vi "Hysteresis.vi"(0 "Max":dbl=4.0 min=-5.0 max=5.0 format="%.3f", 1 "Min":dbl=-4.0 min=-5.0 max=5.0 format="%.3f", 2 "?":bool, 3 "SubVI":bool, 4 "Pattern":string(combo)="0", 5 "?":bool, 6 "Min":dbl=-4.0 min=-10.5 max=10.5 format="%.3f", 7 "Max":dbl=4.0 min=-10.5 max=10.5 format="%.3f", 8 "Amplitude":dbl=2.0 min=1e-09 max=2.0 format="%.3f", 10 "Frequency":dbl=4.0 min=0.001 max=2500000.0 format="%.3g", 13 "?":bool, 14 "Loop":dbl=1.0 min=1.0 step=1.0 format="%#_4g", 16 "Steps":dbl=15.0 min=1.0 step=1.0 format="%#_4g", 18 "Bias Time":dbl=1.0 min=0.0 format="%.4f") -> (12 "Total Loop Time":dbl=40.0 min=0.0 format="%.4f")   [LabVIEW 2016]
uses:
  <vilib>/Utility/file.llb/Write Delimited Spreadsheet (DBL).vi
  <instrlib>/Stanford Research SR865/Stanford Research SR865.lvlib
panel:
  in  "Save As Path":path
  in  "Save As Path":path
  in  "Save As Path":path
  in  "Save As Path":path
  in  "Save As Path":path
  in  "Save As Path":path
  in  "Save As Path":path
  out "Output3-Time":cluster{dbl[], dbl[]}(graph)
  out "Output3-Potential Difference":cluster{dbl[], dbl[]}(graph)
  out "Output2-Time":cluster{dbl[], dbl[]}(graph)
  out "Potential Difference-Time":cluster{dbl[], dbl[]}(graph)
  out "Output1-Time":cluster{dbl[], dbl[]}(graph)
  out "Output1-Potential Difference":cluster{dbl[], dbl[]}(graph)
  out "Output2-Potential Difference":cluster{dbl[], dbl[]}(graph)
  in  "Output 3":i32(ring) items=["None"=-1, "X output"=0, "Y output"=1, "R output"=2, "Theta output"=3, "Aux In 1"=4, "Aux In 2"=5, "Aux In 3"=6, "Aux In 4"=7, "Aux Out 1"=8, "Aux Out 2"=9, "Xnoise"=10, "Ynoise"=11, "Reference Phase"=12, "Sine Out Amplitude"=13, "DC Level"=14, "Int. Ref. Frequency"=15, "Ext. Ref. Frequency"=16]
  in  "Aux Channel":u16(ring)=1 items=["Aux Output 1"=1, "Aux Output 2"=2, "Aux Output 3"=3, "Aux Output 4"=4]
  in  "Output 2":i32(ring)=3 items=["X output", "Y output", "R output", "Theta output", "Aux In 1", "Aux In 2", "Aux In 3", "Aux In 4", "Aux Out 1", "Aux Out 2", "Xnoise", "Ynoise", "Reference Phase", "Sine Out Amplitude", "DC Level", "Int. Ref. Frequency", "Ext. Ref. Frequency"]
  in  "Output 1":i32(ring)=2 items=["X output", "Y output", "R output", "Theta output", "Aux In 1", "Aux In 2", "Aux In 3", "Aux In 4", "Aux Out 1", "Aux Out 2", "Xnoise", "Ynoise", "Reference Phase", "Sine Out Amplitude", "DC Level", "Int. Ref. Frequency", "Ext. Ref. Frequency"]
  in  "Bias Intermission":dbl=0.25 min=0.0 format="%.4f"
  in  "0 V Intermission":dbl=0.25 min=0.0 format="%.4f"
  in  "0 V Time":dbl=1.0 min=0.0 format="%.4f"
  out "VISA resource name out":refnum<visa-resource-name>
  out "error out":errorcluster
  in  "VISA resource name":refnum<visa-resource-name>="LIA"
  in  "error in (no error)":errorcluster
  out "Step Time":dbl=2.5 format="%#.4g"
  # "Configure"
  # "Sine Out DC"
  # "V"
  # "V"
  # "Sine Out AC"
  # "V"
  # "Hz"
  # "Aux Out DC Sawtooth"
  # "V"
  # "V"
  # "Times"
  # "times"
  # "s"
  # "s"
  # "s"
  # "s"
  # "s"
  # "s"
  # "Outputs"
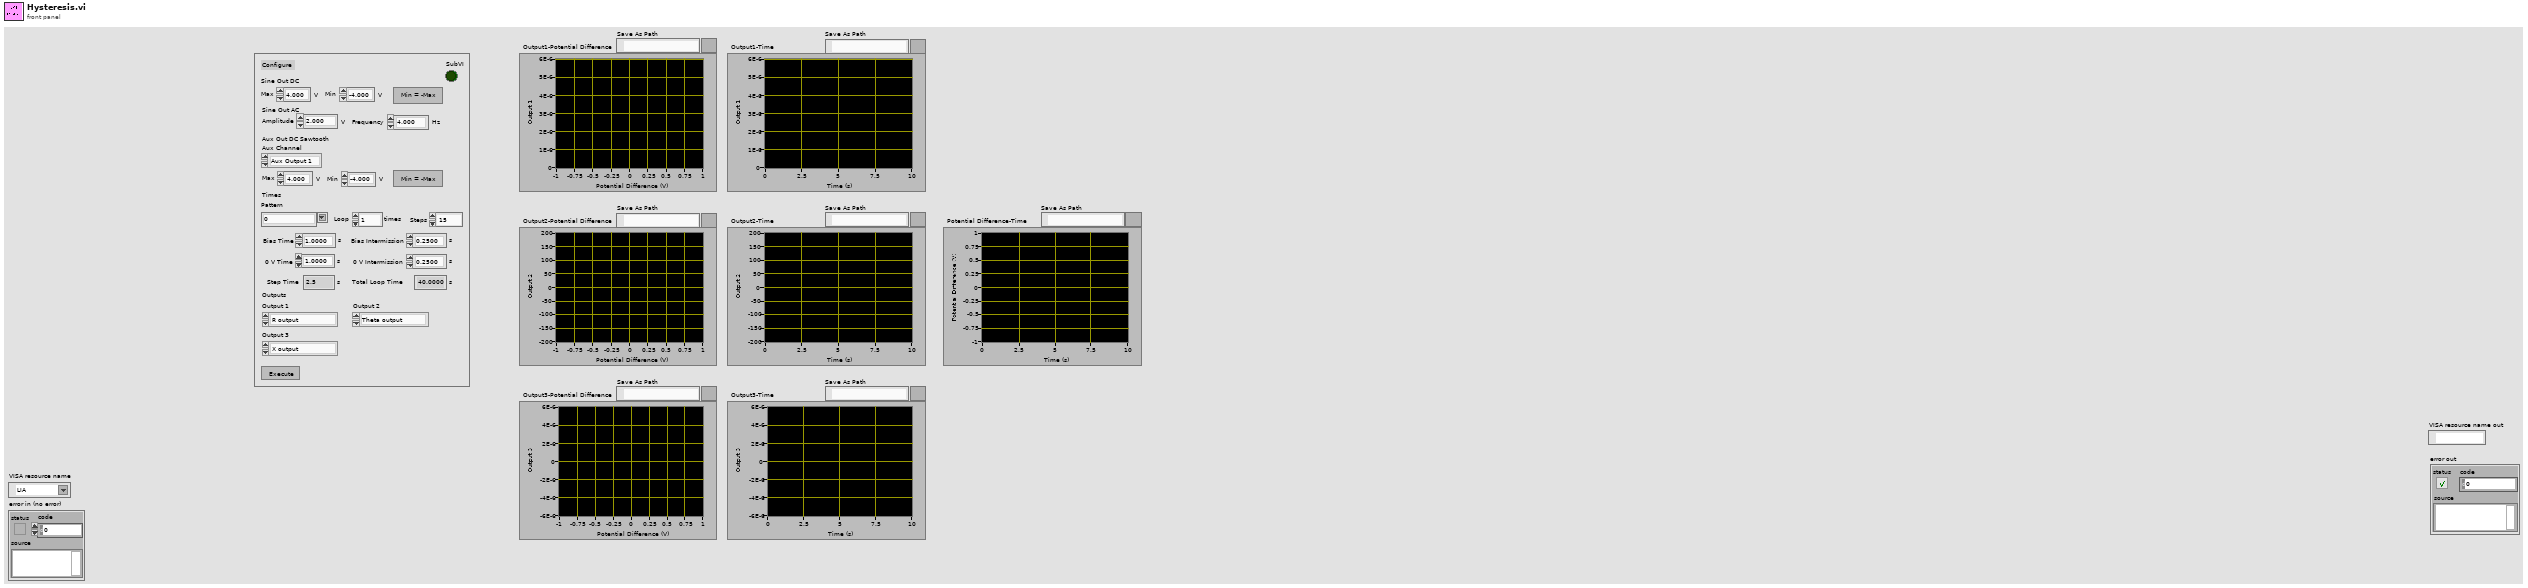
[diagram p1: front panel]
types:
  T1 = cluster{"Value 1":dbl, "Value 2":dbl, "Value 3":dbl}
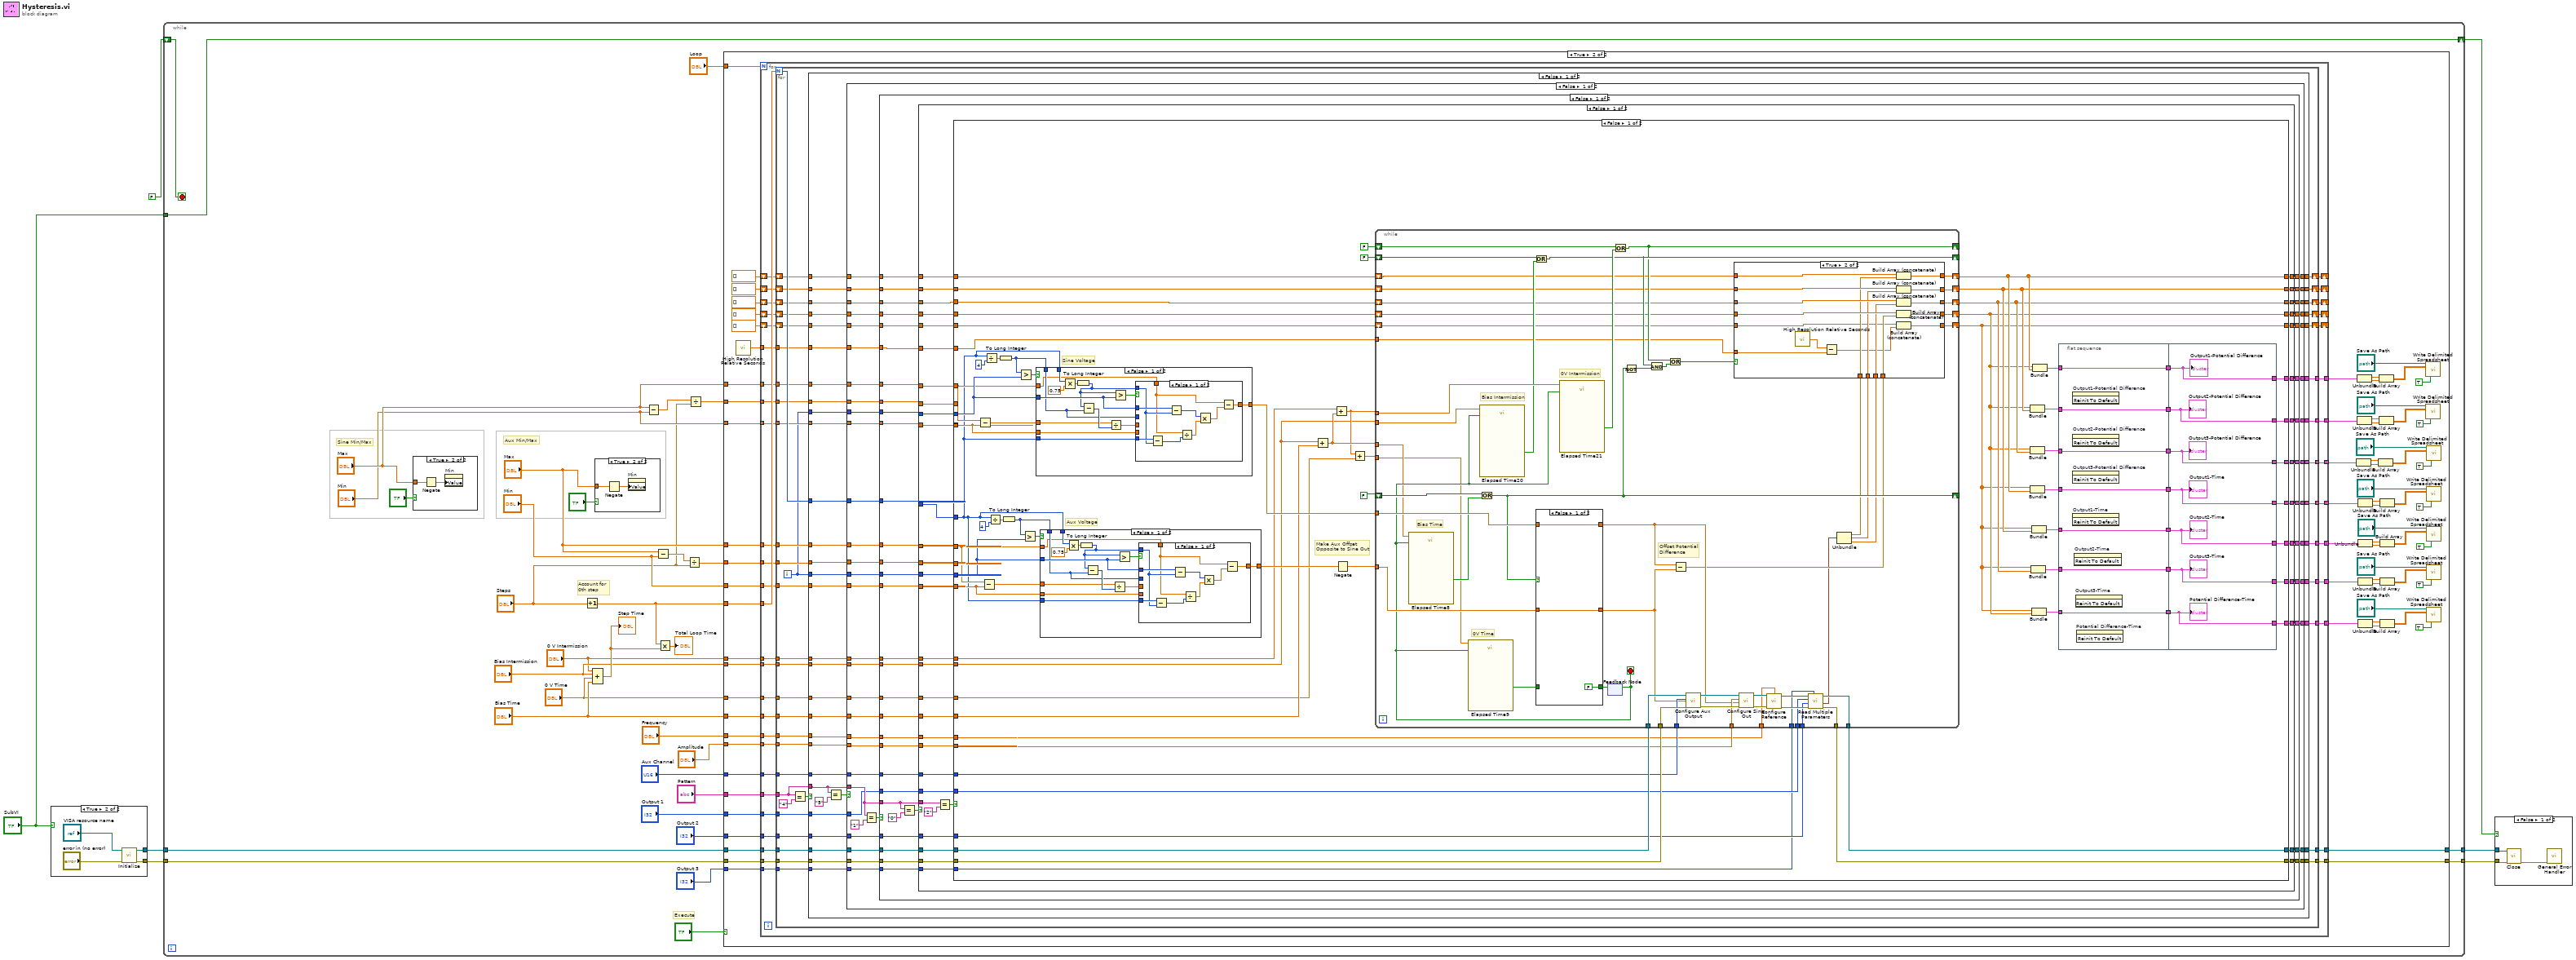
[diagram p0: block diagram]
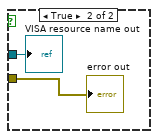
[diagram p2: hidden frame]
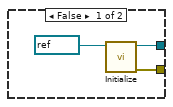
[diagram p3: hidden frame]
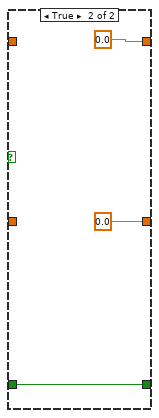
[diagram p6: hidden frame]
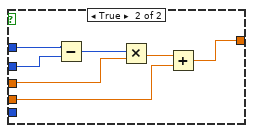
[diagram p7: hidden frame]
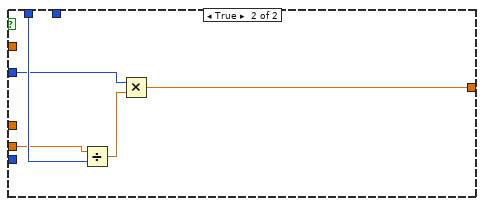
[diagram p8: hidden frame]
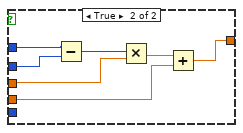
[diagram p9: hidden frame]
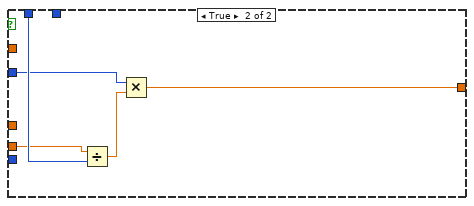
[diagram p10: hidden frame]
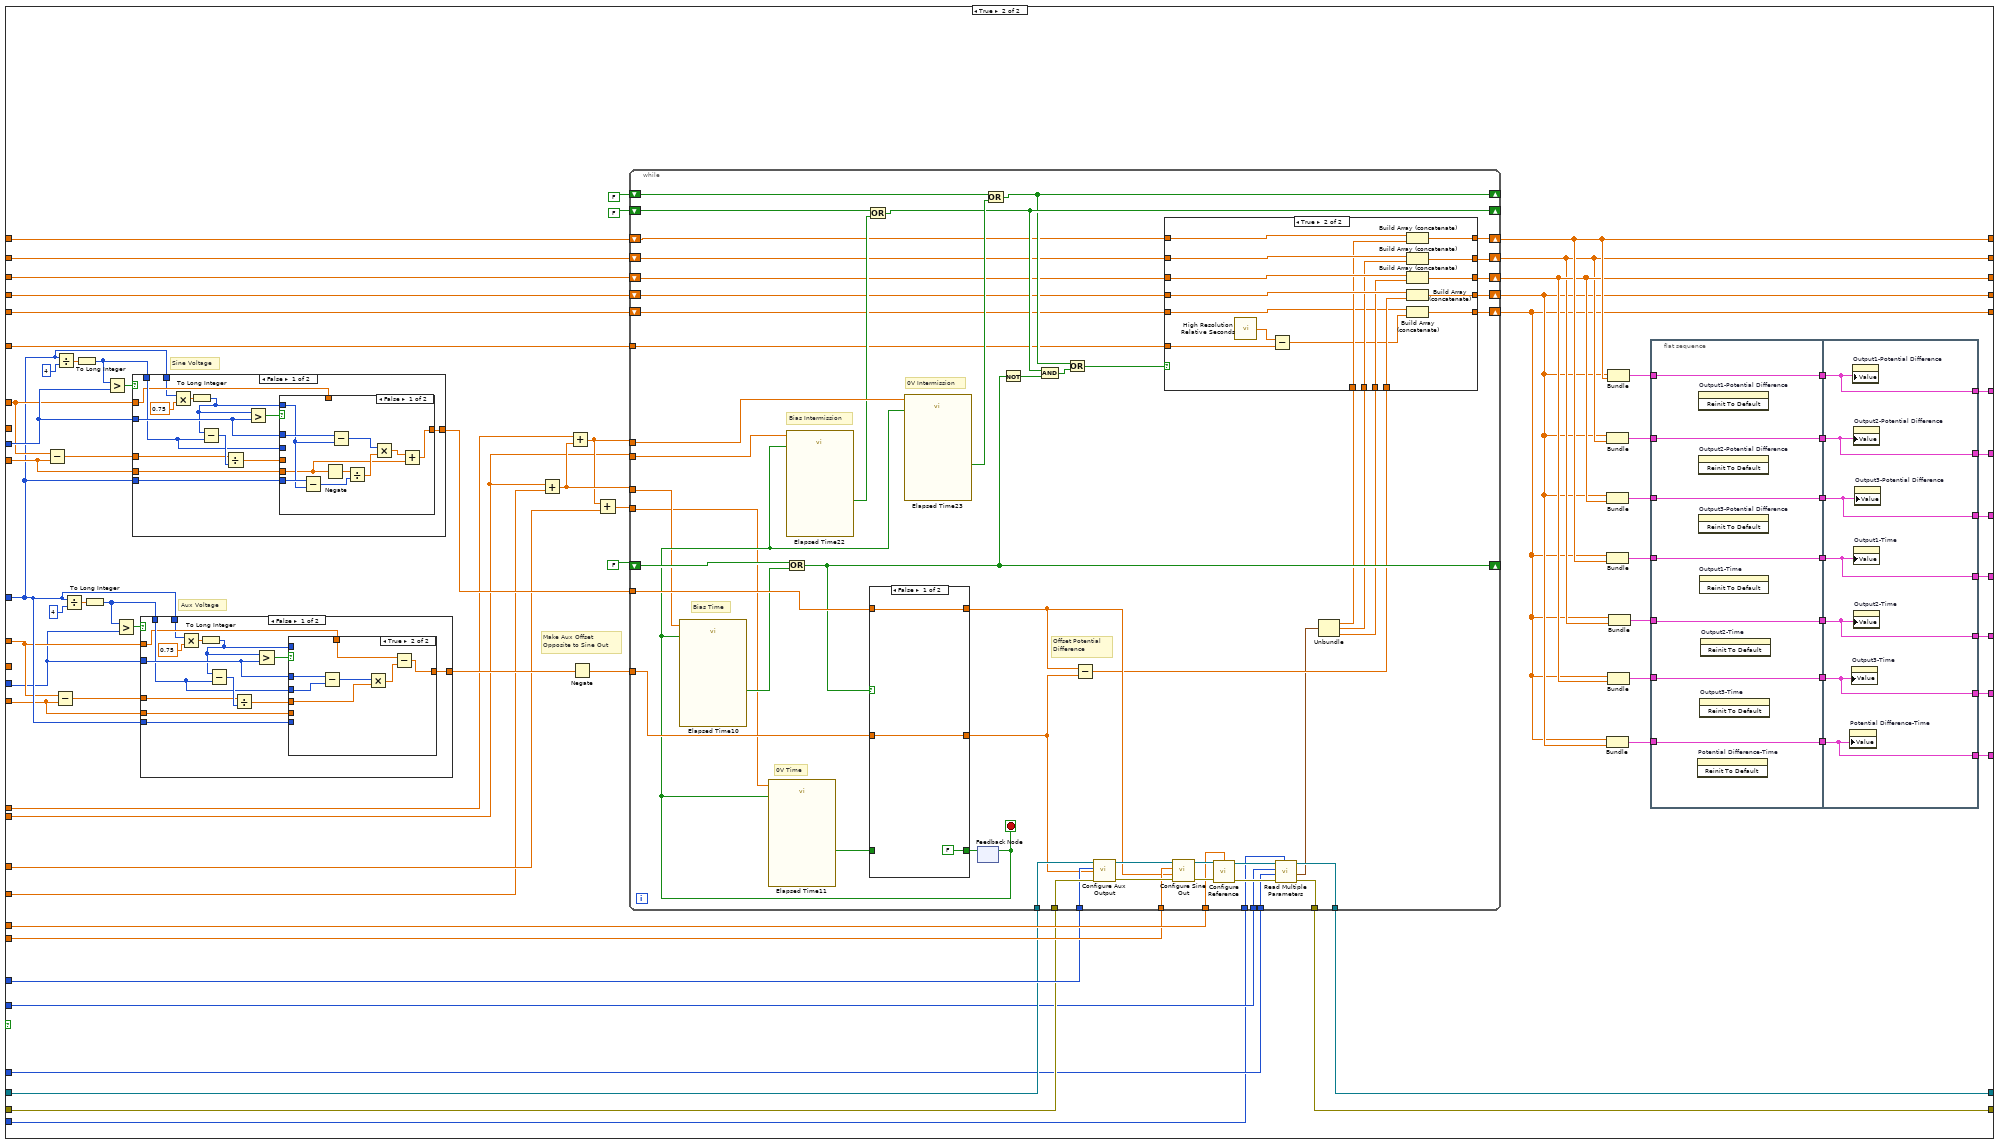
[diagram p11: hidden frame]
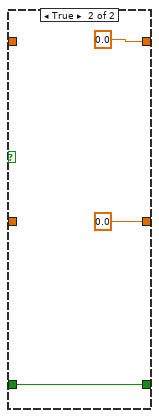
[diagram p13: hidden frame]
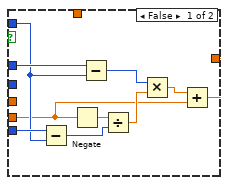
[diagram p14: hidden frame]
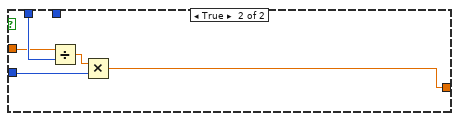
[diagram p15: hidden frame]
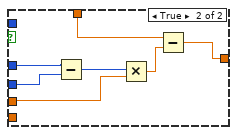
[diagram p16: hidden frame]
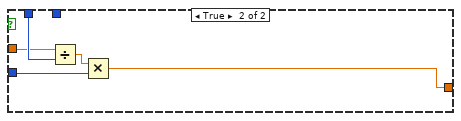
[diagram p17: hidden frame]
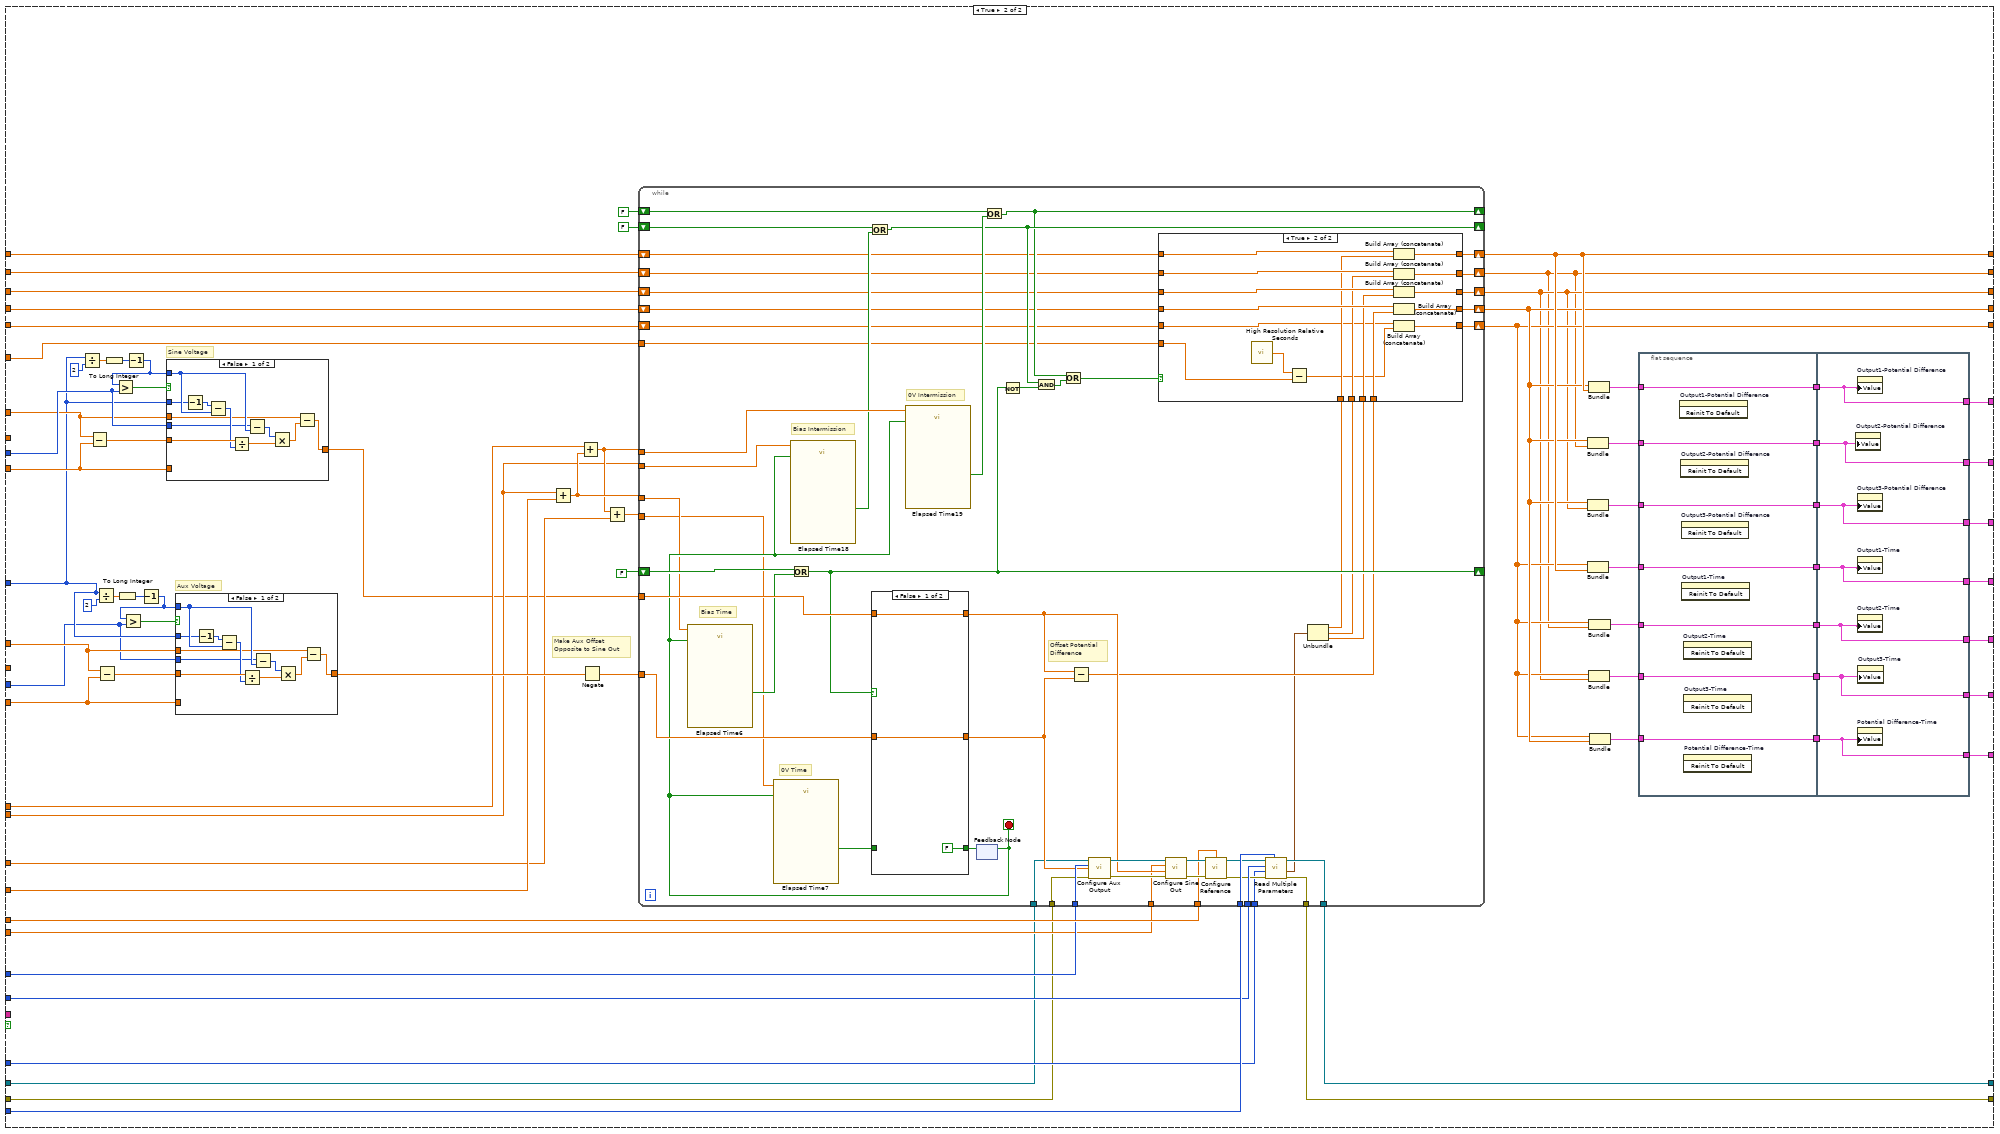
[diagram p18: hidden frame]
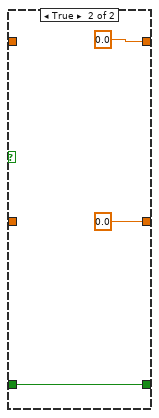
[diagram p20: hidden frame]
diagram:
  n1 = case shown="True" "SubVI" {
    tunnel: [w9 w14] -> w6
    tunnel: [w8 w13] -> w5
    frame False {
      n2 = call <instrlib>:"Initialize.vi"("VISA resource name"=refnum<visa-resource-name> "LIA") -> ("error out"=w8:errorcluster, "VISA resource name out"=w9:refnum<visa-resource-name>)  [unwired: 9 in]
    }
    frame True {
      n3 = call <instrlib>:"Initialize.vi"("error in (no error)"="error in (no error)", "VISA resource name"="VISA resource name") -> ("error out"=w13:errorcluster, "VISA resource name out"=w14:refnum<visa-resource-name>)  [unwired: 8 in]
    }
  }
  n4 = while {
    shift-right: [w26] -> w2
    shift-left: FALSE ("Boolean") -> [w31]
    tunnel: w6 -> [w30]
    tunnel: w5 -> [w29]
    tunnel: [w28] -> w3
    tunnel: [w27] -> w4
    tunnel: "SubVI" -> [w26]
    stop <- w31 stop-if-true
    # "Execute"
    # "Account for\n0th step"
    # "Aux Min/Max"
    # "Sine Min/Max"
    n5 = case shown="True" "?" {
      tunnel: "Max" -> [_ w1597]
      frame False {
      }
      frame True {
        n6 = Negate(x=w1597) -> (-x=w1596:dbl)
        n7 = property on="Min" class="DigNum (strict)"("Value"=w1596) -> ()  [unwired: 2 in, 2 out]
      }
    }
    n8 = Increment(x="Steps") -> (x+1=w20:dbl)
    n9 = Compound Arithmetic op=ADD("0 V Intermission", "Bias Intermission", "0 V Time", "Bias Time") -> (w19:dbl)
    "Step Time" <- w19
    n10 = case shown="True" "?" {
      tunnel: "Max" -> [_ w1595]
      frame False {
      }
      frame True {
        n11 = Negate(x=w1595) -> (-x=w1594:dbl)
        n12 = property on="Min" class="DigNum (strict)"("Value"=w1594) -> ()  [unwired: 2 in, 2 out]
      }
    }
    n13 = Subtract(x="Max", y="Min") -> (x-y=w39:dbl)
    n14 = Subtract(x="Max", y="Min") -> (x-y=w42:dbl)
    n15 = Multiply(x=w20, y=w19) -> (x*y=→"Total Loop Time":dbl)
    n16 = Divide(x=w42, y="Steps") -> (x/y=w44:dbl)
    n17 = Divide(x=w39, y="Steps") -> (x/y=w38:dbl)
    n18 = case shown="True" "?" {
      tunnel: "Loop" -> [_ w120]
      tunnel: w44 -> [_ w119]
      tunnel: "0 V Time" -> [_ w118]
      tunnel: "Pattern" -> [_ w117]
      tunnel: "Frequency" -> [_ w116]
      tunnel: "Amplitude" -> [_ w115]
      tunnel: "Bias Time" -> [_ w114]
      tunnel: w38 -> [_ w113]
      tunnel: w20 -> [_ w112]
      tunnel: "Max" -> [_ w111]
      tunnel: "Min" -> [_ w110]
      tunnel: "Min" -> [_ w109]
      tunnel: "Max" -> [_ w108]
      tunnel: w30 -> [w49 w107]
      tunnel: w29 -> [w48 w106]
      tunnel: [w48 w105] -> w28
      tunnel: [w49 w104] -> w27
      tunnel: "Output 1" -> [_ w103]
      tunnel: "Output 2" -> [_ w102]
      tunnel: "Aux Channel" -> [_ w101]
      tunnel: "Bias Intermission" -> [_ w100]
      tunnel: "0 V Intermission" -> [_ w99]
      tunnel: "Output 3" -> [_ w98]
      frame False {
      }
      frame True {
        n19 = call <vilib>:"High Resolution Relative Seconds.vi"() -> ("relative seconds"=w92:dbl)
        n20 = for {
          N: w120 -> [_]
          tunnel: w112 -> [w160]
          tunnel: w119 -> [w159]
          tunnel: w114 -> [w158]
          tunnel: w118 -> [w157]
          tunnel: w108 -> [w156]
          tunnel: w109 -> [w155]
          tunnel: w117 -> [w154]
          tunnel: w116 -> [w153]
          tunnel: w115 -> [w152]
          tunnel: w113 -> [w151]
          tunnel: w111 -> [w150]
          tunnel: w110 -> [w149]
          tunnel: w107 -> [w148]
          tunnel: w106 -> [w147]
          tunnel: [w146] -> w105
          tunnel: [w145] -> w104
          tunnel: w103 -> [w144]
          tunnel: w102 -> [w143]
          tunnel: w101 -> [w142]
          tunnel: w100 -> [w141]
          tunnel: w99 -> [w140]
          shift-right: [w136] -> _
          shift-left: dbl[] [] -> [w139]
          shift-right: [w135] -> _
          shift-left: dbl[] [] -> [w138]
          shift-right: [w134] -> _
          shift-left: dbl[] [] -> [w137]
          tunnel: w98 -> [w133]
          shift-right: [w132] -> _
          shift-left: dbl[] [] -> [w130]
          shift-right: [w131] -> _
          shift-left: dbl[] [] -> [w129]
          tunnel: w92 -> [w128]
          tunnel: [w127] -> w88
          tunnel: [w126] -> w83
          tunnel: [w125] -> w78
          tunnel: [w124] -> w73
          tunnel: [w123] -> w68
          tunnel: [w122] -> w63
          tunnel: [w121] -> w58
          n21 = for {
            N: w160 -> [w198]
            tunnel: w159 -> [w203]
            tunnel: w158 -> [w202]
            tunnel: w157 -> [w201]
            tunnel: w156 -> [w200]
            tunnel: w155 -> [w199]
            tunnel: w154 -> [w195]
            tunnel: w153 -> [w194]
            tunnel: w152 -> [w193]
            tunnel: w151 -> [w192]
            tunnel: w150 -> [w191]
            tunnel: w149 -> [w190]
            tunnel: w148 -> [w188]
            tunnel: w147 -> [w187]
            tunnel: [w186] -> w146
            tunnel: [w185] -> w145
            tunnel: w144 -> [w184]
            tunnel: w143 -> [w183]
            tunnel: w142 -> [w182]
            tunnel: w141 -> [w181]
            tunnel: w140 -> [w180]
            shift-right: [w179] -> w136
            shift-left: w139 -> [w174]
            shift-right: [w178] -> w135
            shift-left: w138 -> [w175]
            shift-right: [w177] -> w134
            shift-left: w137 -> [w176]
            tunnel: w133 -> [w173]
            shift-right: [w172] -> w132
            shift-left: w130 -> [w170]
            shift-right: [w171] -> w131
            shift-left: w129 -> [w169]
            tunnel: w128 -> [w168]
            tunnel: [w167] -> w127
            tunnel: [w166] -> w126
            tunnel: [w165] -> w125
            tunnel: [w164] -> w124
            tunnel: [w163] -> w123
            tunnel: [w162] -> w122
            tunnel: [w161] -> w121
            i -> [w189]
            n22 = Equal?(x=w195, y="4") -> (x = y?=w196:bool)
            n23 = case shown="False" w196 {
              tunnel: w203 -> [w242 w1493]
              tunnel: w189 -> [w243 w1496]
              tunnel: w202 -> [w244 w1453]
              tunnel: w201 -> [w245 w1454]
              tunnel: w195 -> [w240 _]
              tunnel: w200 -> [w241 _]
              tunnel: w199 -> [w238 w1494]
              tunnel: w198 -> [w239 _]
              tunnel: w194 -> [w237 w1465]
              tunnel: w193 -> [w236 w1464]
              tunnel: w192 -> [w235 w1491]
              tunnel: w191 -> [w233 _]
              tunnel: w190 -> [w232 w1489]
              tunnel: w189 -> [w234 w1490]
              tunnel: w188 -> [w231 w1461]
              tunnel: w187 -> [w230 w1462]
              tunnel: [w229 w1466] -> w186
              tunnel: [w228 w1467] -> w185
              tunnel: w184 -> [w224 w1459]
              tunnel: w183 -> [w223 w1458]
              tunnel: w182 -> [w222 w1463]
              tunnel: w181 -> [w220 w1456]
              tunnel: w180 -> [w221 w1457]
              tunnel: [w219 w1442] -> w179
              tunnel: [w218 w1441] -> w178
              tunnel: [w217 w1443] -> w177
              tunnel: w176 -> [w225 w1450]
              tunnel: w175 -> [w226 w1449]
              tunnel: w174 -> [w227 w1448]
              tunnel: w173 -> [w216 w1460]
              tunnel: [w215 w1444] -> w172
              tunnel: [w214 w1445] -> w171
              tunnel: w170 -> [w213 w1451]
              tunnel: w169 -> [w212 w1452]
              tunnel: w168 -> [w211 w1446]
              tunnel: [w210 w1440] -> w167
              tunnel: [w209 w1434] -> w166
              tunnel: [w208 w1435] -> w165
              tunnel: [w207 w1436] -> w164
              tunnel: [w206 w1437] -> w163
              tunnel: [w205 w1438] -> w162
              tunnel: [w204 w1439] -> w161
              frame False {
                n24 = Equal?(x=w240, y="5") -> (x = y?=w246:bool)
                n25 = case shown="False" w246 {
                  tunnel: w245 -> [w289 w1300]
                  tunnel: w244 -> [w288 w1301]
                  tunnel: w243 -> [w286 w1336]
                  tunnel: w242 -> [w284 w1335]
                  tunnel: w241 -> [w283 w1333]
                  tunnel: w240 -> [w282 _]
                  tunnel: w239 -> [w287 _]
                  tunnel: w238 -> [w285 _]
                  tunnel: w237 -> [w280 w1311]
                  tunnel: w236 -> [w281 w1312]
                  tunnel: w235 -> [w277 w1331]
                  tunnel: w234 -> [w278 w1330]
                  tunnel: w233 -> [w276 w1329]
                  tunnel: w232 -> [w279 _]
                  tunnel: w231 -> [w275 w1313]
                  tunnel: w230 -> [w274 w1314]
                  tunnel: [w273 w1307] -> w229
                  tunnel: [w272 w1306] -> w228
                  tunnel: w227 -> [w266 w1294]
                  tunnel: w226 -> [w267 w1295]
                  tunnel: w225 -> [w268 w1296]
                  tunnel: w224 -> [w262 w1309]
                  tunnel: w223 -> [w261 w1308]
                  tunnel: w222 -> [w263 w1305]
                  tunnel: w221 -> [w265 w1304]
                  tunnel: w220 -> [w264 w1303]
                  tunnel: [w269 w1284] -> w219
                  tunnel: [w270 w1283] -> w218
                  tunnel: [w271 w1282] -> w217
                  tunnel: w216 -> [w260 w1310]
                  tunnel: [w259 w1286] -> w215
                  tunnel: [w258 w1285] -> w214
                  tunnel: w213 -> [w257 w1297]
                  tunnel: w212 -> [w256 w1298]
                  tunnel: w211 -> [w255 w1281]
                  tunnel: [w254 w1280] -> w210
                  tunnel: [w253 w1274] -> w209
                  tunnel: [w252 w1275] -> w208
                  tunnel: [w251 w1276] -> w207
                  tunnel: [w250 w1277] -> w206
                  tunnel: [w249 w1278] -> w205
                  tunnel: [w248 w1279] -> w204
                  frame False {
                    n26 = Equal?(x=w282, y="1") -> (x = y?=w290:bool)
                    n27 = case shown="False" w290 {
                      tunnel: w289 -> [w335 w1103]
                      tunnel: w288 -> [w334 w1104]
                      tunnel: w287 -> [w329 w1129]
                      tunnel: w286 -> [w332 w1128]
                      tunnel: w285 -> [w333 w1127]
                      tunnel: w284 -> [w331 _]
                      tunnel: w283 -> [w330 w1126]
                      tunnel: w282 -> [w326 _]
                      tunnel: w281 -> [w324 w1099]
                      tunnel: w280 -> [w325 w1100]
                      tunnel: w279 -> [w320 w1134]
                      tunnel: w278 -> [w321 w1135]
                      tunnel: w277 -> [w322 _]
                      tunnel: w276 -> [w323 w1136]
                      tunnel: w275 -> [w319 w1096]
                      tunnel: w274 -> [w318 w1097]
                      tunnel: [w317 w1095] -> w273
                      tunnel: [w316 w1094] -> w272
                      tunnel: [w307 w1074] -> w271
                      tunnel: [w306 w1075] -> w270
                      tunnel: [w305 w1076] -> w269
                      tunnel: w268 -> [w310 w1089]
                      tunnel: w267 -> [w309 w1090]
                      tunnel: w266 -> [w308 w1091]
                      tunnel: w265 -> [w312 w1101]
                      tunnel: w264 -> [w311 w1102]
                      tunnel: w263 -> [w315 w1098]
                      tunnel: w262 -> [w314 w1106]
                      tunnel: w261 -> [w313 w1107]
                      tunnel: w260 -> [w304 w1105]
                      tunnel: [w303 w1077] -> w259
                      tunnel: [w302 w1078] -> w258
                      tunnel: w257 -> [w301 w1088]
                      tunnel: w256 -> [w300 w1087]
                      tunnel: w255 -> [w299 w1086]
                      tunnel: [w298 w1073] -> w254
                      tunnel: [w297 w1067] -> w253
                      tunnel: [w296 w1068] -> w252
                      tunnel: [w295 w1069] -> w251
                      tunnel: [w294 w1070] -> w250
                      tunnel: [w293 w1071] -> w249
                      tunnel: [w292 w1072] -> w248
                      frame False {
                        n28 = Equal?(x=w326, y="0") -> (x = y?=w327:bool)
                        n29 = case shown="False" w327 {
                          tunnel: w335 -> [w375 w896]
                          tunnel: w334 -> [w376 w897]
                          tunnel: w333 -> [w370 w924]
                          tunnel: w332 -> [w374 w921]
                          tunnel: w331 -> [w373 _]
                          tunnel: w330 -> [w372 w923]
                          tunnel: w329 -> [w371 w922]
                          tunnel: w326 -> [w378 _]
                          tunnel: w325 -> [w369 w889]
                          tunnel: w324 -> [w368 w885]
                          tunnel: w323 -> [w365 w928]
                          tunnel: w322 -> [w366 _]
                          tunnel: w321 -> [w367 w929]
                          tunnel: w320 -> [w364 w930]
                          tunnel: w319 -> [w363 w880]
                          tunnel: w318 -> [w362 w881]
                          tunnel: [w361 w887] -> w317
                          tunnel: [w360 w886] -> w316
                          tunnel: w315 -> [w357 w888]
                          tunnel: w314 -> [w356 w883]
                          tunnel: w313 -> [w355 w882]
                          tunnel: w312 -> [w359 w899]
                          tunnel: w311 -> [w358 w898]
                          tunnel: w310 -> [w351 w894]
                          tunnel: w309 -> [w349 w893]
                          tunnel: w308 -> [w350 w892]
                          tunnel: [w354 w868] -> w307
                          tunnel: [w353 w867] -> w306
                          tunnel: [w352 w871] -> w305
                          tunnel: w304 -> [w348 w884]
                          tunnel: [w347 w870] -> w303
                          tunnel: [w346 w869] -> w302
                          tunnel: w301 -> [w345 w891]
                          tunnel: w300 -> [w344 w890]
                          tunnel: w299 -> [w343 w879]
                          tunnel: [w342 w866] -> w298
                          tunnel: [w341 w860] -> w297
                          tunnel: [w340 w861] -> w296
                          tunnel: [w339 w862] -> w295
                          tunnel: [w338 w863] -> w294
                          tunnel: [w337 w864] -> w293
                          tunnel: [w336 w865] -> w292
                          frame False {
                            n30 = Equal?(x=w378, y="2") -> (x = y?=w377:bool)
                            n31 = case shown="False" w377 {
                              tunnel: w376 -> [w423 w650]
                              tunnel: w375 -> [w422 w651]
                              tunnel: w374 -> [w437 w674]
                              tunnel: w373 -> [_ _]
                              tunnel: w372 -> [w436 w676]
                              tunnel: w371 -> [w435 w677]
                              tunnel: w370 -> [w438 w675]
                              tunnel: w369 -> [w415 w649]
                              tunnel: w368 -> [w416 w648]
                              tunnel: w364 -> [w446 w685]
                              tunnel: w367 -> [w445 w688]
                              tunnel: w366 -> [_ _]
                              tunnel: w365 -> [w444 w686]
                              tunnel: w364 -> [_ _]
                              tunnel: w363 -> [w421 w645]
                              tunnel: w362 -> [w420 w646]
                              tunnel: [w419 w641] -> w361
                              tunnel: [w418 w640] -> w360
                              tunnel: w359 -> [w425 w653]
                              tunnel: w358 -> [w424 w652]
                              tunnel: w357 -> [w417 w647]
                              tunnel: w356 -> [w414 w643]
                              tunnel: w355 -> [w413 w644]
                              tunnel: [w390 w631] -> w354
                              tunnel: [w391 w630] -> w353
                              tunnel: [w392 w632] -> w352
                              tunnel: w351 -> [w411 w655]
                              tunnel: w350 -> [w409 w657]
                              tunnel: w349 -> [w410 w656]
                              tunnel: w348 -> [w412 w642]
                              tunnel: [w389 w629] -> w347
                              tunnel: [w388 w628] -> w346
                              tunnel: w345 -> [w408 w654]
                              tunnel: w344 -> [w400 w627]
                              tunnel: w343 -> [w387 w626]
                              tunnel: [w386 w625] -> w342
                              tunnel: [w385 w619] -> w341
                              tunnel: [w384 w620] -> w340
                              tunnel: [w383 w621] -> w339
                              tunnel: [w382 w622] -> w338
                              tunnel: [w381 w623] -> w337
                              tunnel: [w380 w624] -> w336
                              frame False {
                                # "Make Aux Offset \nOpposite to Sine Out"
                                # "Aux Voltage"
                                # "Sine Voltage"
                                n32 = Subtract(x=w444, y=w446) -> (x-y=w449:dbl)
                                n33 = Subtract(x=w436, y=w438) -> (x-y=w441:dbl)
                                n34 = Divide(x=w435, y=4) -> (x/y=w448:dbl)
                                n35 = Divide(x=w435, y=4) -> (x/y=w440:dbl)
                                n36 = To Long Integer(number=w448) -> (32bit integer=w447:i32)
                                n37 = To Long Integer(number=w440) -> (32bit integer=w439:i32)
                                n38 = Greater?(x=w447, y=w445) -> (0:w451:bool)
                                n39 = Greater?(x=w439, y=w437) -> (0:w443:bool)
                                n40 = case shown="False" w451 {
                                tunnel: [w590 w617] -> w426
                                tunnel: w447 -> [w591 w618]
                                tunnel: w445 -> [w595 w615]
                                tunnel: w449 -> [w592 _]
                                tunnel: w435 -> [w589 _]
                                tunnel: w446 -> [w588 w614]
                                tunnel: w435 -> [w587 _]
                                tunnel: w444 -> [w584 _]
                                frame False {
                                n41 = Multiply(x=w587, y=0.75) -> (x*y=w586:dbl)
                                n42 = To Long Integer(number=w586) -> (32bit integer=w585:i32)
                                n43 = Subtract(x=w585, y=w591) -> (x-y=w593:i32)
                                n44 = Divide(x=w592, y=w593) -> (x/y=w594:dbl)
                                n45 = Greater?(x=w585, y=w595) -> (0:w596:bool)
                                n46 = case shown="False" w596 {
                                tunnel: w585 -> [w603 _]
                                tunnel: w595 -> [w604 w613]
                                tunnel: w594 -> [_ w611]
                                tunnel: w591 -> [_ w612]
                                tunnel: [w598 w607] -> w590
                                tunnel: w589 -> [w606 _]
                                tunnel: w588 -> [_ w608]
                                tunnel: w584 -> [w600 _]
                                frame False {
                                n47 = Subtract(x=w606, y=w603) -> (x-y=w605:i32)
                                n48 = Subtract(x=w604, y=w603) -> (x-y=w601:i32)
                                n49 = Divide(x=w600, y=w605) -> (x/y=w602:dbl)
                                n50 = Multiply(x=w601, y=w602) -> (x*y=w599:dbl)
                                n51 = Subtract(x=w600, y=w599) -> (x-y=w598:dbl)
                                }
                                frame True {
                                n52 = Subtract(x=w613, y=w612) -> (x-y=w610:i32)
                                n53 = Multiply(x=w610, y=w611) -> (x*y=w609:dbl)
                                n54 = Add(x=w609, y=w608) -> (x+y=w607:dbl)
                                }
                                }
                                }
                                frame True {
                                n55 = Divide(x=w614, y=w618) -> (x/y=w616:dbl)
                                n56 = Multiply(x=w615, y=w616) -> (x*y=w617:dbl)
                                }
                                }
                                n57 = case shown="False" w443 {
                                tunnel: [w555 w582] -> w427
                                tunnel: w439 -> [w556 w583]
                                tunnel: w437 -> [w560 w580]
                                tunnel: w441 -> [w557 _]
                                tunnel: w435 -> [w554 _]
                                tunnel: w438 -> [w553 w579]
                                tunnel: w435 -> [w552 _]
                                tunnel: w436 -> [w549 _]
                                frame False {
                                n58 = Multiply(x=w552, y=0.75) -> (x*y=w551:dbl)
                                n59 = To Long Integer(number=w551) -> (32bit integer=w550:i32)
                                n60 = Subtract(x=w550, y=w556) -> (x-y=w558:i32)
                                n61 = Divide(x=w557, y=w558) -> (x/y=w559:dbl)
                                n62 = Greater?(x=w550, y=w560) -> (0:w561:bool)
                                n63 = case shown="False" w561 {
                                tunnel: w550 -> [w568 _]
                                tunnel: w560 -> [w569 w578]
                                tunnel: w559 -> [_ w576]
                                tunnel: w556 -> [_ w577]
                                tunnel: [w563 w572] -> w555
                                tunnel: w554 -> [w571 _]
                                tunnel: w553 -> [_ w573]
                                tunnel: w549 -> [w565 _]
                                frame False {
                                n64 = Subtract(x=w571, y=w568) -> (x-y=w570:i32)
                                n65 = Subtract(x=w569, y=w568) -> (x-y=w566:i32)
                                n66 = Divide(x=w565, y=w570) -> (x/y=w567:dbl)
                                n67 = Multiply(x=w566, y=w567) -> (x*y=w564:dbl)
                                n68 = Subtract(x=w565, y=w564) -> (x-y=w563:dbl)
                                }
                                frame True {
                                n69 = Subtract(x=w578, y=w577) -> (x-y=w575:i32)
                                n70 = Multiply(x=w575, y=w576) -> (x*y=w574:dbl)
                                n71 = Add(x=w574, y=w573) -> (x+y=w572:dbl)
                                }
                                }
                                }
                                frame True {
                                n72 = Divide(x=w579, y=w583) -> (x/y=w581:dbl)
                                n73 = Multiply(x=w580, y=w581) -> (x*y=w582:dbl)
                                }
                                }
                                n74 = Add(x=w424, y=w423) -> (x+y=w431:dbl)
                                n75 = Add(x=w425, y=w431) -> (x+y=w429:dbl)
                                n76 = Negate(x=w427) -> (-x=w428:dbl)
                                n77 = Add(x=w429, y=w422) -> (x+y=w430:dbl)
                                n78 = while {
                                tunnel: w428 -> [w520]
                                tunnel: w430 -> [w492]
                                tunnel: w426 -> [w519]
                                shift-right: [w491] -> _
                                shift-left: FALSE -> [w518]
                                tunnel: w421 -> [w514]
                                tunnel: w420 -> [w513]
                                tunnel: [w504] -> w418
                                tunnel: [w503] -> w419
                                tunnel: w416 -> [w510]
                                tunnel: w415 -> [w507]
                                tunnel: w414 -> [w502]
                                tunnel: w413 -> [w501]
                                tunnel: w417 -> [w500]
                                shift-right: [w487] -> _
                                shift-left: FALSE -> [w495]
                                shift-right: [w488] -> _
                                shift-left: FALSE -> [w497]
                                tunnel: w424 -> [w498]
                                tunnel: w431 -> [w494]
                                tunnel: w429 -> [w493]
                                shift-right: [w483] -> w392
                                shift-left: w409 -> [w480]
                                shift-right: [w482] -> w391
                                shift-left: w410 -> [w479]
                                shift-right: [w481] -> w390
                                shift-left: w411 -> [w478]
                                tunnel: w412 -> [w473]
                                shift-right: [w470] -> w389
                                shift-left: w408 -> [w468]
                                shift-right: [w469] -> w388
                                shift-left: w400 -> [w467]
                                tunnel: w387 -> [w466]
                                stop <- w499 stop-if-true
                                # "Offset Potential\nDifference"
                                # "0V Intermission"
                                # "Bias Intermission"
                                # "0V Time"
                                # "Bias Time"
                                n79 = feedback #1() -> (w499:bool)  [unwired: 1 in]
                                n80 = call "Elapsed Time8"("Time Target (s)"=w494, "Reset"=w499) -> ("Time has Elapsed"=w517:bool)  [unwired: 10 in, 7 out]
                                n81 = call "Elapsed Time9"("Time Target (s)"=w492, "Reset"=w499) -> ("Time has Elapsed"=w515:bool)  [unwired: 10 in, 7 out]
                                n82 = call "Elapsed Time20"("Time Target (s)"=w498, "Reset"=w499) -> ("Time has Elapsed"=w490:bool)  [unwired: 10 in, 7 out]
                                n83 = Or(x=w518, y=w517) -> (x .or. y?=w491:bool)
                                n84 = Or(x=w497, y=w490) -> (x .or. y?=w488:bool)
                                n85 = case shown="False" w491 {
                                tunnel: [w543 0.0] -> w485
                                tunnel: [w545 0.0] -> w484
                                tunnel: w520 -> [w545 _]
                                tunnel: [FALSE ("Time has Elapsed") w546] -> w516
                                tunnel: w519 -> [w543 _]
                                tunnel: w515 -> [_ w546]
                                frame False {
                                }
                                frame True {
                                }
                                }
                                n86 = call "Elapsed Time21"("Time Target (s)"=w493, "Reset"=w499) -> ("Time has Elapsed"=w496:bool)  [unwired: 10 in, 7 out]
                                n87 = feedback-in #1(w516) -> ()
                                n88 = Or(x=w495, y=w496) -> (x .or. y?=w487:bool)
                                n89 = Not(x=w491) -> (.not. x?=w489:bool)
                                n90 = And(x=w488, y=w489) -> (x .and. y?=w486:bool)
                                n91 = Or(x=w487, y=w486) -> (x .or. y?=w474:bool)
                                n92 = Subtract(x=w485, y=w484) -> (x-y=w475:dbl)
                                n93 = call <instrlib>:"Configure Aux Output.vi"("error in (no error)"=w513, "Aux Output Voltage (0)"=w484, "Aux Channel (1: Channel 1)"=w500, "VISA resource name"=w514) -> ("error out"=w511:errorcluster, "VISA resource name out"=w512:refnum<visa-resource-name>)  [unwired: 6 in]
                                n94 = call <instrlib>:"Configure Sine Out.vi"("error in (no error)"=w511, "Sine Out DC Level to Voltage (0 V)"=w485, "Sine Out Amplitude to Voltage (0 V)"=w510, "VISA resource name"=w512) -> ("error out"=w508:errorcluster, "VISA resource name out"=w509:refnum<visa-resource-name>)  [unwired: 6 in]
                                n95 = call <instrlib>:"Configure Reference.vi"("VISA resource name"=w509, "Internal Reference Frequency (100000Hz)"=w507, "error in (no error)"=w508) -> ("VISA resource name out"=w506:refnum<visa-resource-name>, "error out"=w505:errorcluster)  [unwired: 11 in]
                                n96 = call <instrlib>:"Read Multiple Parameters.vi"("Single Lock-in Parameter 3 (-1: None)"=w473, "error in (no error)"=w505, "Single Lock-in Parameter 2 (0: X output)"=w501, "Single Lock-in Parameter 1 (0: X output)"=w502, "VISA resource name"=w506) -> ("error out"=w503:errorcluster, "Output Value(3 parameters)"=w472:T1, "VISA resource name out"=w504:refnum<visa-resource-name>)  [unwired: 3 in, 1 out]
                                n97 = Unbundle(w472) -> ("Value 1"=w477:dbl, "Value 2"=w476:dbl, "Value 3"=w471:dbl)
                                n98 = case shown="True" w474 {
                                tunnel: [w525 w542] -> w483
                                tunnel: [w524 w541] -> w482
                                tunnel: [w523 w540] -> w481
                                tunnel: w480 -> [w525 w539]
                                tunnel: w479 -> [w524 w538]
                                tunnel: w478 -> [w523 w537]
                                tunnel: w477 -> [_ w530]
                                tunnel: w476 -> [_ w531]
                                tunnel: w475 -> [_ w533]
                                tunnel: w471 -> [_ w532]
                                tunnel: [w522 w536] -> w470
                                tunnel: [w521 w535] -> w469
                                tunnel: w468 -> [w522 w534]
                                tunnel: w467 -> [w521 w529]
                                tunnel: w466 -> [_ w528]
                                frame False {
                                }
                                frame True {
                                n99 = call <vilib>:"High Resolution Relative Seconds.vi"() -> ("relative seconds"=w527:dbl)
                                n100 = Subtract(x=w527, y=w528) -> (x-y=w526:dbl)
                                n101 = Build Array (concatenate)(w539, w530) -> (w542:dbl[])
                                n102 = Build Array (concatenate)(w538, w531) -> (w541:dbl[])
                                n103 = Build Array (concatenate)(w537, w532) -> (w540:dbl[])
                                n104 = Build Array (concatenate)(w534, w533) -> (w536:dbl[])
                                n105 = Build Array (concatenate)(w529, w526) -> (w535:dbl[])
                                }
                                }
                                }
                                n106 = Bundle(w389, w391) -> (w398:cluster{dbl[], dbl[]})  [unwired: 1 in]
                                n107 = Bundle(w389, w390) -> (w397:cluster{dbl[], dbl[]})  [unwired: 1 in]
                                n108 = Bundle(w388, w392) -> (w396:cluster{dbl[], dbl[]})  [unwired: 1 in]
                                n109 = Bundle(w388, w390) -> (w394:cluster{dbl[], dbl[]})  [unwired: 1 in]
                                n110 = Bundle(w388, w391) -> (w395:cluster{dbl[], dbl[]})  [unwired: 1 in]
                                n111 = Bundle(w388, w389) -> (w393:cluster{dbl[], dbl[]})  [unwired: 1 in]
                                n112 = Bundle(w389, w392) -> (w399:cluster{dbl[], dbl[]})  [unwired: 1 in]
                                n113 = flat-sequence {
                                tunnel: [w458] -> w407
                                tunnel: w399 -> [w458]
                                tunnel: [w457] -> w406
                                tunnel: w398 -> [w457]
                                tunnel: w393 -> [w456]
                                tunnel: [w456] -> w405
                                tunnel: w394 -> [w455]
                                tunnel: [w455] -> w404
                                tunnel: w395 -> [w454]
                                tunnel: [w454] -> w403
                                tunnel: w397 -> [w453]
                                tunnel: [w453] -> w402
                                tunnel: w396 -> [w452]
                                tunnel: [w452] -> w401
                                tunnel: w407 -> [w464]
                                tunnel: w406 -> [w463]
                                tunnel: w405 -> [w465]
                                tunnel: w404 -> [w459]
                                tunnel: w403 -> [w460]
                                tunnel: w402 -> [w462]
                                tunnel: w401 -> [w461]
                                tunnel: [w465] -> w386
                                tunnel: [w464] -> w385
                                tunnel: [w463] -> w384
                                tunnel: [w462] -> w383
                                tunnel: [w461] -> w382
                                tunnel: [w460] -> w381
                                tunnel: [w459] -> w380
                                frame #0 {
                                n114 = invoke on="Output1-Potential Difference" class="XYGraph (strict)" method="Reinit To Default"() -> ()  [unwired: 3 in, 3 out]
                                n115 = invoke on="Output2-Potential Difference" class="XYGraph (strict)" method="Reinit To Default"() -> ()  [unwired: 3 in, 3 out]
                                n116 = invoke on="Output3-Potential Difference" class="XYGraph (strict)" method="Reinit To Default"() -> ()  [unwired: 3 in, 3 out]
                                n117 = invoke on="Output1-Time" class="XYGraph (strict)" method="Reinit To Default"() -> ()  [unwired: 3 in, 3 out]
                                n118 = invoke on="Output2-Time" class="XYGraph (strict)" method="Reinit To Default"() -> ()  [unwired: 3 in, 3 out]
                                n119 = invoke on="Output3-Time" class="XYGraph (strict)" method="Reinit To Default"() -> ()  [unwired: 3 in, 3 out]
                                n120 = invoke on="Potential Difference-Time" class="XYGraph (strict)" method="Reinit To Default"() -> ()  [unwired: 3 in, 3 out]
                                }
                                frame #1 {
                                "Output1-Potential Difference" <- w464
                                "Output2-Potential Difference" <- w463
                                "Output3-Potential Difference" <- w462
                                "Output1-Time" <- w461
                                "Output2-Time" <- w460
                                "Output3-Time" <- w459
                                "Potential Difference-Time" <- w465
                                }
                                }
                              }
                              frame True {
                                # "Make Aux Offset \nOpposite to Sine Out"
                                # "Aux Voltage"
                                # "Sine Voltage"
                                n121 = Subtract(x=w686, y=w685) -> (x-y=w687:dbl)
                                n122 = Subtract(x=w676, y=w675) -> (x-y=w680:dbl)
                                n123 = Divide(x=w677, y=4) -> (x/y=w684:dbl)
                                n124 = Divide(x=w677, y=4) -> (x/y=w679:dbl)
                                n125 = To Long Integer(number=w684) -> (32bit integer=w683:i32)
                                n126 = To Long Integer(number=w679) -> (32bit integer=w678:i32)
                                n127 = Greater?(x=w683, y=w688) -> (0:w690:bool)
                                n128 = Greater?(x=w678, y=w674) -> (0:w682:bool)
                                n129 = case shown="False" w690 {
                                tunnel: [w829 w855] -> w659
                                tunnel: w683 -> [w831 w859]
                                tunnel: w688 -> [w835 w856]
                                tunnel: w687 -> [w832 _]
                                tunnel: w686 -> [w830 w858]
                                tunnel: w677 -> [w828 _]
                                tunnel: w685 -> [w827 _]
                                tunnel: w677 -> [w826 _]
                                frame False {
                                n130 = Multiply(x=w826, y=0.75) -> (x*y=w825:dbl)
                                n131 = To Long Integer(number=w825) -> (32bit integer=w824:i32)
                                n132 = Subtract(x=w824, y=w831) -> (x-y=w833:i32)
                                n133 = Divide(x=w832, y=w833) -> (x/y=w834:dbl)
                                n134 = Greater?(x=w824, y=w835) -> (0:w836:bool)
                                n135 = case shown="False" w836 {
                                tunnel: w824 -> [w843 _]
                                tunnel: w835 -> [w844 w854]
                                tunnel: w834 -> [_ w851]
                                tunnel: w831 -> [_ w853]
                                tunnel: w830 -> [_ w852]
                                tunnel: [w838 w848] -> w829
                                tunnel: w828 -> [w847 _]
                                tunnel: w827 -> [w839 _]
                                frame False {
                                n136 = Subtract(x=w847, y=w843) -> (x-y=w845:i32)
                                n137 = Negate(x=w839) -> (-x=w846:dbl)
                                n138 = Subtract(x=w844, y=w843) -> (x-y=w841:i32)
                                n139 = Divide(x=w846, y=w845) -> (x/y=w842:dbl)
                                n140 = Multiply(x=w841, y=w842) -> (x*y=w840:dbl)
                                n141 = Add(x=w840, y=w839) -> (x+y=w838:dbl)
                                }
                                frame True {
                                n142 = Subtract(x=w854, y=w853) -> (x-y=w850:i32)
                                n143 = Multiply(x=w850, y=w851) -> (x*y=w849:dbl)
                                n144 = Subtract(x=w852, y=w849) -> (x-y=w848:dbl)
                                }
                                }
                                }
                                frame True {
                                n145 = Divide(x=w858, y=w859) -> (x/y=w857:dbl)
                                n146 = Multiply(x=w857, y=w856) -> (x*y=w855:dbl)
                                }
                                }
                                n147 = case shown="False" w682 {
                                tunnel: [w793 w819] -> w658
                                tunnel: w678 -> [w795 w823]
                                tunnel: w674 -> [w799 w820]
                                tunnel: w680 -> [w796 _]
                                tunnel: w676 -> [w794 w822]
                                tunnel: w677 -> [w792 _]
                                tunnel: w675 -> [w791 _]
                                tunnel: w677 -> [w790 _]
                                frame False {
                                n148 = Multiply(x=w790, y=0.75) -> (x*y=w789:dbl)
                                n149 = To Long Integer(number=w789) -> (32bit integer=w788:i32)
                                n150 = Subtract(x=w788, y=w795) -> (x-y=w797:i32)
                                n151 = Divide(x=w796, y=w797) -> (x/y=w798:dbl)
                                n152 = Greater?(x=w788, y=w799) -> (0:w800:bool)
                                n153 = case shown="True" w800 {
                                tunnel: w788 -> [w807 _]
                                tunnel: w799 -> [w808 w818]
                                tunnel: w798 -> [_ w815]
                                tunnel: w795 -> [_ w817]
                                tunnel: w794 -> [_ w816]
                                tunnel: [w802 w812] -> w793
                                tunnel: w792 -> [w811 _]
                                tunnel: w791 -> [w803 _]
                                frame False {
                                n154 = Subtract(x=w811, y=w807) -> (x-y=w809:i32)
                                n155 = Negate(x=w803) -> (-x=w810:dbl)
                                n156 = Subtract(x=w808, y=w807) -> (x-y=w805:i32)
                                n157 = Divide(x=w810, y=w809) -> (x/y=w806:dbl)
                                n158 = Multiply(x=w805, y=w806) -> (x*y=w804:dbl)
                                n159 = Add(x=w804, y=w803) -> (x+y=w802:dbl)
                                }
                                frame True {
                                n160 = Subtract(x=w818, y=w817) -> (x-y=w814:i32)
                                n161 = Multiply(x=w814, y=w815) -> (x*y=w813:dbl)
                                n162 = Subtract(x=w816, y=w813) -> (x-y=w812:dbl)
                                }
                                }
                                }
                                frame True {
                                n163 = Divide(x=w822, y=w823) -> (x/y=w821:dbl)
                                n164 = Multiply(x=w821, y=w820) -> (x*y=w819:dbl)
                                }
                                }
                                n165 = Add(x=w652, y=w650) -> (x+y=w663:dbl)
                                n166 = Add(x=w653, y=w663) -> (x+y=w661:dbl)
                                n167 = Negate(x=w658) -> (-x=w660:dbl)
                                n168 = Add(x=w661, y=w651) -> (x+y=w662:dbl)
                                n169 = while {
                                tunnel: w660 -> [w759]
                                tunnel: w662 -> [w731]
                                tunnel: w659 -> [w758]
                                shift-right: [w730] -> _
                                shift-left: FALSE -> [w757]
                                tunnel: w645 -> [w753]
                                tunnel: w646 -> [w752]
                                tunnel: [w743] -> w640
                                tunnel: [w742] -> w641
                                tunnel: w648 -> [w749]
                                tunnel: w649 -> [w746]
                                tunnel: w643 -> [w741]
                                tunnel: w644 -> [w740]
                                tunnel: w647 -> [w739]
                                shift-right: [w726] -> _
                                shift-left: FALSE -> [w734]
                                shift-right: [w727] -> _
                                shift-left: FALSE -> [w736]
                                tunnel: w652 -> [w737]
                                tunnel: w663 -> [w733]
                                tunnel: w661 -> [w732]
                                shift-right: [w722] -> w632
                                shift-left: w657 -> [w719]
                                shift-right: [w721] -> w630
                                shift-left: w656 -> [w718]
                                shift-right: [w720] -> w631
                                shift-left: w655 -> [w717]
                                tunnel: w642 -> [w712]
                                shift-right: [w709] -> w629
                                shift-left: w654 -> [w707]
                                shift-right: [w708] -> w628
                                shift-left: w627 -> [w706]
                                tunnel: w626 -> [w705]
                                stop <- w738 stop-if-true
                                # "Offset Potential\nDifference"
                                # "0V Intermission"
                                # "Bias Intermission"
                                # "0V Time"
                                # "Bias Time"
                                n170 = feedback #2() -> (w738:bool)  [unwired: 1 in]
                                n171 = call "Elapsed Time10"("Time Target (s)"=w733, "Reset"=w738) -> ("Time has Elapsed"=w756:bool)  [unwired: 10 in, 7 out]
                                n172 = call "Elapsed Time11"("Time Target (s)"=w731, "Reset"=w738) -> ("Time has Elapsed"=w754:bool)  [unwired: 10 in, 7 out]
                                n173 = call "Elapsed Time22"("Time Target (s)"=w737, "Reset"=w738) -> ("Time has Elapsed"=w729:bool)  [unwired: 10 in, 7 out]
                                n174 = Or(x=w757, y=w756) -> (x .or. y?=w730:bool)
                                n175 = Or(x=w736, y=w729) -> (x .or. y?=w727:bool)
                                n176 = case shown="False" w730 {
                                tunnel: [w782 0.0] -> w724
                                tunnel: [w784 0.0] -> w723
                                tunnel: w759 -> [w784 _]
                                tunnel: [FALSE ("Time has Elapsed") w785] -> w755
                                tunnel: w758 -> [w782 _]
                                tunnel: w754 -> [_ w785]
                                frame False {
                                }
                                frame True {
                                }
                                }
                                n177 = call "Elapsed Time23"("Time Target (s)"=w732, "Reset"=w738) -> ("Time has Elapsed"=w735:bool)  [unwired: 10 in, 7 out]
                                n178 = feedback-in #2(w755) -> ()
                                n179 = Or(x=w734, y=w735) -> (x .or. y?=w726:bool)
                                n180 = Not(x=w730) -> (.not. x?=w728:bool)
                                n181 = And(x=w727, y=w728) -> (x .and. y?=w725:bool)
                                n182 = Or(x=w726, y=w725) -> (x .or. y?=w713:bool)
                                n183 = Subtract(x=w724, y=w723) -> (x-y=w714:dbl)
                                n184 = call <instrlib>:"Configure Aux Output.vi"("error in (no error)"=w752, "Aux Output Voltage (0)"=w723, "Aux Channel (1: Channel 1)"=w739, "VISA resource name"=w753) -> ("error out"=w750:errorcluster, "VISA resource name out"=w751:refnum<visa-resource-name>)  [unwired: 6 in]
                                n185 = call <instrlib>:"Configure Sine Out.vi"("error in (no error)"=w750, "Sine Out DC Level to Voltage (0 V)"=w724, "Sine Out Amplitude to Voltage (0 V)"=w749, "VISA resource name"=w751) -> ("error out"=w747:errorcluster, "VISA resource name out"=w748:refnum<visa-resource-name>)  [unwired: 6 in]
                                n186 = call <instrlib>:"Configure Reference.vi"("VISA resource name"=w748, "Internal Reference Frequency (100000Hz)"=w746, "error in (no error)"=w747) -> ("VISA resource name out"=w745:refnum<visa-resource-name>, "error out"=w744:errorcluster)  [unwired: 11 in]
                                n187 = call <instrlib>:"Read Multiple Parameters.vi"("Single Lock-in Parameter 3 (-1: None)"=w712, "error in (no error)"=w744, "Single Lock-in Parameter 2 (0: X output)"=w740, "Single Lock-in Parameter 1 (0: X output)"=w741, "VISA resource name"=w745) -> ("error out"=w742:errorcluster, "Output Value(3 parameters)"=w711:T1, "VISA resource name out"=w743:refnum<visa-resource-name>)  [unwired: 3 in, 1 out]
                                n188 = Unbundle(w711) -> ("Value 1"=w716:dbl, "Value 2"=w715:dbl, "Value 3"=w710:dbl)
                                n189 = case shown="True" w713 {
                                tunnel: [w764 w781] -> w722
                                tunnel: [w763 w780] -> w721
                                tunnel: [w762 w779] -> w720
                                tunnel: w719 -> [w764 w778]
                                tunnel: w718 -> [w763 w777]
                                tunnel: w717 -> [w762 w776]
                                tunnel: w716 -> [_ w769]
                                tunnel: w715 -> [_ w770]
                                tunnel: w714 -> [_ w772]
                                tunnel: w710 -> [_ w771]
                                tunnel: [w761 w775] -> w709
                                tunnel: [w760 w774] -> w708
                                tunnel: w707 -> [w761 w773]
                                tunnel: w706 -> [w760 w768]
                                tunnel: w705 -> [_ w766]
                                frame False {
                                }
                                frame True {
                                n190 = call <vilib>:"High Resolution Relative Seconds.vi"() -> ("relative seconds"=w765:dbl)
                                n191 = Subtract(x=w765, y=w766) -> (x-y=w767:dbl)
                                n192 = Build Array (concatenate)(w778, w769) -> (w781:dbl[])
                                n193 = Build Array (concatenate)(w777, w770) -> (w780:dbl[])
                                n194 = Build Array (concatenate)(w776, w771) -> (w779:dbl[])
                                n195 = Build Array (concatenate)(w773, w772) -> (w775:dbl[])
                                n196 = Build Array (concatenate)(w768, w767) -> (w774:dbl[])
                                }
                                }
                                }
                                n197 = Bundle(w628, w629) -> (w639:cluster{dbl[], dbl[]})  [unwired: 1 in]
                                n198 = Bundle(w629, w630) -> (w634:cluster{dbl[], dbl[]})  [unwired: 1 in]
                                n199 = Bundle(w629, w631) -> (w635:cluster{dbl[], dbl[]})  [unwired: 1 in]
                                n200 = Bundle(w628, w632) -> (w636:cluster{dbl[], dbl[]})  [unwired: 1 in]
                                n201 = Bundle(w629, w632) -> (w633:cluster{dbl[], dbl[]})  [unwired: 1 in]
                                n202 = Bundle(w628, w631) -> (w638:cluster{dbl[], dbl[]})  [unwired: 1 in]
                                n203 = Bundle(w628, w630) -> (w637:cluster{dbl[], dbl[]})  [unwired: 1 in]
                                n204 = flat-sequence {
                                tunnel: [w697] -> w673
                                tunnel: w633 -> [w697]
                                tunnel: [w696] -> w672
                                tunnel: w634 -> [w696]
                                tunnel: w639 -> [w695]
                                tunnel: [w695] -> w671
                                tunnel: w638 -> [w694]
                                tunnel: [w694] -> w670
                                tunnel: w637 -> [w693]
                                tunnel: [w693] -> w669
                                tunnel: w635 -> [w692]
                                tunnel: [w692] -> w668
                                tunnel: w636 -> [w691]
                                tunnel: [w691] -> w667
                                tunnel: w673 -> [w698]
                                tunnel: w672 -> [w699]
                                tunnel: w671 -> [w704]
                                tunnel: w670 -> [w703]
                                tunnel: w669 -> [w702]
                                tunnel: w668 -> [w700]
                                tunnel: w667 -> [w701]
                                tunnel: [w704] -> w625
                                tunnel: [w703] -> w624
                                tunnel: [w702] -> w623
                                tunnel: [w701] -> w622
                                tunnel: [w700] -> w621
                                tunnel: [w699] -> w620
                                tunnel: [w698] -> w619
                                frame #0 {
                                n205 = invoke on="Potential Difference-Time" class="XYGraph (strict)" method="Reinit To Default"() -> ()  [unwired: 3 in, 3 out]
                                n206 = invoke on="Output1-Potential Difference" class="XYGraph (strict)" method="Reinit To Default"() -> ()  [unwired: 3 in, 3 out]
                                n207 = invoke on="Output2-Potential Difference" class="XYGraph (strict)" method="Reinit To Default"() -> ()  [unwired: 3 in, 3 out]
                                n208 = invoke on="Output3-Potential Difference" class="XYGraph (strict)" method="Reinit To Default"() -> ()  [unwired: 3 in, 3 out]
                                n209 = invoke on="Output1-Time" class="XYGraph (strict)" method="Reinit To Default"() -> ()  [unwired: 3 in, 3 out]
                                n210 = invoke on="Output3-Time" class="XYGraph (strict)" method="Reinit To Default"() -> ()  [unwired: 3 in, 3 out]
                                n211 = invoke on="Output2-Time" class="XYGraph (strict)" method="Reinit To Default"() -> ()  [unwired: 3 in, 3 out]
                                }
                                frame #1 {
                                n212 = property on="Potential Difference-Time" class="XYGraph (strict)"("Value"=w704) -> ()  [unwired: 2 in, 2 out]
                                n213 = property on="Output3-Time" class="XYGraph (strict)"("Value"=w703) -> ()  [unwired: 2 in, 2 out]
                                n214 = property on="Output1-Potential Difference" class="XYGraph (strict)"("Value"=w698) -> ()  [unwired: 2 in, 2 out]
                                n215 = property on="Output2-Potential Difference" class="XYGraph (strict)"("Value"=w699) -> ()  [unwired: 2 in, 2 out]
                                n216 = property on="Output1-Time" class="XYGraph (strict)"("Value"=w701) -> ()  [unwired: 2 in, 2 out]
                                n217 = property on="Output2-Time" class="XYGraph (strict)"("Value"=w702) -> ()  [unwired: 2 in, 2 out]
                                n218 = property on="Output3-Potential Difference" class="XYGraph (strict)"("Value"=w700) -> ()  [unwired: 2 in, 2 out]
                                }
                                }
                              }
                            }
                          }
                          frame True {
                            # "Make Aux Offset \nOpposite to Sine Out"
                            # "Aux Voltage"
                            # "Sine Voltage"
                            n219 = Divide(x=w922, y=2) -> (x/y=w920:dbl)
                            n220 = Subtract(x=w928, y=w930) -> (x-y=w931:dbl)
                            n221 = Divide(x=w922, y=2) -> (x/y=w919:dbl)
                            n222 = Subtract(x=w923, y=w924) -> (x-y=w925:dbl)
                            n223 = To Long Integer(number=w920) -> (32bit integer=w918:i32)
                            n224 = To Long Integer(number=w919) -> (32bit integer=w916:i32)
                            n225 = Decrement(x=w918) -> (x-1=w917:i32)
                            n226 = Greater?(x=w917, y=w929) -> (0:w932:bool)
                            n227 = Decrement(x=w916) -> (x-1=w915:i32)
                            n228 = Greater?(x=w915, y=w921) -> (0:w926:bool)
                            n229 = case shown="False" w932 {
                              tunnel: w931 -> [w1059 w1066]
                              tunnel: w917 -> [w1057 w1065]
                              tunnel: w930 -> [_ w1061]
                              tunnel: w929 -> [w1051 w1063]
                              tunnel: [w1052 w1060] -> w895
                              tunnel: w922 -> [w1049 _]
                              tunnel: w928 -> [w1053 _]
                              frame False {
                                n230 = Decrement(x=w1049) -> (x-1=w1050:i32)
                                n231 = Subtract(x=w1050, y=w1057) -> (x-y=w1058:i32)
                                n232 = Divide(x=w1059, y=w1058) -> (x/y=w1055:dbl)
                                n233 = Subtract(x=w1051, y=w1057) -> (x-y=w1056:i32)
                                n234 = Multiply(x=w1056, y=w1055) -> (x*y=w1054:dbl)
                                n235 = Subtract(x=w1053, y=w1054) -> (x-y=w1052:dbl)
                              }
                              frame True {
                                n236 = Divide(x=w1066, y=w1065) -> (x/y=w1064:dbl)
                                n237 = Multiply(x=w1063, y=w1064) -> (x*y=w1062:dbl)
                                n238 = Add(x=w1062, y=w1061) -> (x+y=w1060:dbl)
                              }
                            }
                            n239 = case shown="False" w926 {
                              tunnel: w925 -> [w1041 w1048]
                              tunnel: w915 -> [w1039 w1047]
                              tunnel: w924 -> [_ w1043]
                              tunnel: w921 -> [w1033 w1045]
                              tunnel: [w1034 w1042] -> w900
                              tunnel: w922 -> [w1032 _]
                              tunnel: w923 -> [w1035 _]
                              frame False {
                                n240 = Decrement(x=w1032) -> (x-1=w1031:i32)
                                n241 = Subtract(x=w1031, y=w1039) -> (x-y=w1040:i32)
                                n242 = Divide(x=w1041, y=w1040) -> (x/y=w1037:dbl)
                                n243 = Subtract(x=w1033, y=w1039) -> (x-y=w1038:i32)
                                n244 = Multiply(x=w1038, y=w1037) -> (x*y=w1036:dbl)
                                n245 = Subtract(x=w1035, y=w1036) -> (x-y=w1034:dbl)
                              }
                              frame True {
                                n246 = Divide(x=w1048, y=w1047) -> (x/y=w1046:dbl)
                                n247 = Multiply(x=w1045, y=w1046) -> (x*y=w1044:dbl)
                                n248 = Add(x=w1044, y=w1043) -> (x+y=w1042:dbl)
                              }
                            }
                            n249 = Add(x=w898, y=w897) -> (x+y=w904:dbl)
                            n250 = Add(x=w899, y=w904) -> (x+y=w902:dbl)
                            n251 = Negate(x=w900) -> (-x=w901:dbl)
                            n252 = Add(x=w902, y=w896) -> (x+y=w903:dbl)
                            n253 = while {
                              tunnel: w901 -> [w1002]
                              tunnel: w903 -> [w981]
                              tunnel: w895 -> [w1001]
                              shift-right: [w980] -> _
                              shift-left: FALSE -> [w1000]
                              tunnel: [w991] -> w886
                              tunnel: [w990] -> w887
                              tunnel: w889 -> [w992]
                              tunnel: w888 -> [w989]
                              shift-right: [w976] -> _
                              shift-left: FALSE -> [w984]
                              shift-right: [w977] -> _
                              shift-left: FALSE -> [w986]
                              tunnel: w898 -> [w987]
                              tunnel: w904 -> [w983]
                              tunnel: w902 -> [w982]
                              shift-right: [w972] -> w871
                              shift-left: w892 -> [w969]
                              shift-right: [w971] -> w867
                              shift-left: w893 -> [w968]
                              shift-right: [w970] -> w868
                              shift-left: w894 -> [w967]
                              shift-right: [w960] -> w870
                              shift-left: w891 -> [w958]
                              shift-right: [w959] -> w869
                              shift-left: w890 -> [w957]
                              tunnel: w885 -> [w956]
                              tunnel: w884 -> [w955]
                              tunnel: w883 -> [w954]
                              tunnel: w882 -> [w952]
                              tunnel: w881 -> [w950]
                              tunnel: w880 -> [w949]
                              tunnel: w879 -> [w948]
                              stop <- w988 stop-if-true
                              # "Offset Potential\nDifference"
                              # "0V Intermission"
                              # "Bias Intermission"
                              # "0V Time"
                              # "Bias Time"
                              n254 = feedback #3() -> (w988:bool)  [unwired: 1 in]
                              n255 = call "Elapsed Time6"("Time Target (s)"=w983, "Reset"=w988) -> ("Time has Elapsed"=w999:bool)  [unwired: 10 in, 7 out]
                              n256 = call "Elapsed Time7"("Time Target (s)"=w981, "Reset"=w988) -> ("Time has Elapsed"=w997:bool)  [unwired: 10 in, 7 out]
                              n257 = call "Elapsed Time18"("Time Target (s)"=w987, "Reset"=w988) -> ("Time has Elapsed"=w979:bool)  [unwired: 10 in, 7 out]
                              n258 = Or(x=w1000, y=w999) -> (x .or. y?=w980:bool)
                              n259 = Or(x=w986, y=w979) -> (x .or. y?=w977:bool)
                              n260 = case shown="False" w980 {
                                tunnel: [w1025 0.0] -> w974
                                tunnel: [w1027 0.0] -> w973
                                tunnel: w1002 -> [w1027 _]
                                tunnel: [FALSE ("Time has Elapsed") w1028] -> w998
                                tunnel: w1001 -> [w1025 _]
                                tunnel: w997 -> [_ w1028]
                                frame False {
                                }
                                frame True {
                                }
                              }
                              n261 = call "Elapsed Time19"("Time Target (s)"=w982, "Reset"=w988) -> ("Time has Elapsed"=w985:bool)  [unwired: 10 in, 7 out]
                              n262 = feedback-in #3(w998) -> ()
                              n263 = Or(x=w984, y=w985) -> (x .or. y?=w976:bool)
                              n264 = Not(x=w980) -> (.not. x?=w978:bool)
                              n265 = And(x=w977, y=w978) -> (x .and. y?=w975:bool)
                              n266 = Or(x=w976, y=w975) -> (x .or. y?=w963:bool)
                              n267 = Subtract(x=w974, y=w973) -> (x-y=w964:dbl)
                              n268 = call <instrlib>:"Configure Aux Output.vi"("error in (no error)"=w950, "Aux Output Voltage (0)"=w973, "Aux Channel (1: Channel 1)"=w989, "VISA resource name"=w949) -> ("error out"=w995:errorcluster, "VISA resource name out"=w996:refnum<visa-resource-name>)  [unwired: 6 in]
                              n269 = call <instrlib>:"Configure Sine Out.vi"("error in (no error)"=w995, "Sine Out DC Level to Voltage (0 V)"=w974, "Sine Out Amplitude to Voltage (0 V)"=w956, "VISA resource name"=w996) -> ("error out"=w993:errorcluster, "VISA resource name out"=w994:refnum<visa-resource-name>)  [unwired: 6 in]
                              n270 = call <instrlib>:"Configure Reference.vi"("VISA resource name"=w994, "Internal Reference Frequency (100000Hz)"=w992, "error in (no error)"=w993) -> ("VISA resource name out"=w951:refnum<visa-resource-name>, "error out"=w953:errorcluster)  [unwired: 11 in]
                              n271 = call <instrlib>:"Read Multiple Parameters.vi"("Single Lock-in Parameter 3 (-1: None)"=w955, "error in (no error)"=w953, "Single Lock-in Parameter 2 (0: X output)"=w952, "Single Lock-in Parameter 1 (0: X output)"=w954, "VISA resource name"=w951) -> ("error out"=w990:errorcluster, "Output Value(3 parameters)"=w962:T1, "VISA resource name out"=w991:refnum<visa-resource-name>)  [unwired: 3 in, 1 out]
                              n272 = Unbundle(w962) -> ("Value 1"=w966:dbl, "Value 2"=w965:dbl, "Value 3"=w961:dbl)
                              n273 = case shown="True" w963 {
                                tunnel: [w1007 w1024] -> w972
                                tunnel: [w1006 w1023] -> w971
                                tunnel: [w1005 w1022] -> w970
                                tunnel: w969 -> [w1007 w1021]
                                tunnel: w968 -> [w1006 w1020]
                                tunnel: w967 -> [w1005 w1019]
                                tunnel: w966 -> [_ w1012]
                                tunnel: w965 -> [_ w1013]
                                tunnel: w964 -> [_ w1015]
                                tunnel: w961 -> [_ w1014]
                                tunnel: [w1004 w1018] -> w960
                                tunnel: [w1003 w1017] -> w959
                                tunnel: w958 -> [w1004 w1016]
                                tunnel: w957 -> [w1003 w1011]
                                tunnel: w948 -> [_ w1009]
                                frame False {
                                }
                                frame True {
                                n274 = call <vilib>:"High Resolution Relative Seconds.vi"() -> ("relative seconds"=w1008:dbl)
                                n275 = Subtract(x=w1008, y=w1009) -> (x-y=w1010:dbl)
                                n276 = Build Array (concatenate)(w1021, w1012) -> (w1024:dbl[])
                                n277 = Build Array (concatenate)(w1020, w1013) -> (w1023:dbl[])
                                n278 = Build Array (concatenate)(w1019, w1014) -> (w1022:dbl[])
                                n279 = Build Array (concatenate)(w1016, w1015) -> (w1018:dbl[])
                                n280 = Build Array (concatenate)(w1011, w1010) -> (w1017:dbl[])
                                }
                              }
                            }
                            n281 = Bundle(w870, w867) -> (w875:cluster{dbl[], dbl[]})  [unwired: 1 in]
                            n282 = Bundle(w870, w868) -> (w874:cluster{dbl[], dbl[]})  [unwired: 1 in]
                            n283 = Bundle(w869, w871) -> (w873:cluster{dbl[], dbl[]})  [unwired: 1 in]
                            n284 = Bundle(w870, w871) -> (w876:cluster{dbl[], dbl[]})  [unwired: 1 in]
                            n285 = Bundle(w869, w868) -> (w877:cluster{dbl[], dbl[]})  [unwired: 1 in]
                            n286 = Bundle(w869, w867) -> (w872:cluster{dbl[], dbl[]})  [unwired: 1 in]
                            n287 = Bundle(w869, w870) -> (w878:cluster{dbl[], dbl[]})  [unwired: 1 in]
                            n288 = flat-sequence {
                              tunnel: [w940] -> w914
                              tunnel: w876 -> [w940]
                              tunnel: [w939] -> w913
                              tunnel: w875 -> [w939]
                              tunnel: w878 -> [w938]
                              tunnel: [w938] -> w912
                              tunnel: w877 -> [w937]
                              tunnel: [w937] -> w911
                              tunnel: w872 -> [w936]
                              tunnel: [w936] -> w910
                              tunnel: w874 -> [w935]
                              tunnel: [w935] -> w909
                              tunnel: w873 -> [w934]
                              tunnel: [w934] -> w908
                              tunnel: w914 -> [w941]
                              tunnel: w913 -> [w942]
                              tunnel: w912 -> [w947]
                              tunnel: w911 -> [w946]
                              tunnel: w910 -> [w945]
                              tunnel: w909 -> [w943]
                              tunnel: w908 -> [w944]
                              tunnel: [w947] -> w866
                              tunnel: [w946] -> w865
                              tunnel: [w945] -> w864
                              tunnel: [w944] -> w863
                              tunnel: [w943] -> w862
                              tunnel: [w942] -> w861
                              tunnel: [w941] -> w860
                              frame #0 {
                                n289 = invoke on="Output1-Potential Difference" class="XYGraph (strict)" method="Reinit To Default"() -> ()  [unwired: 3 in, 3 out]
                                n290 = invoke on="Output2-Potential Difference" class="XYGraph (strict)" method="Reinit To Default"() -> ()  [unwired: 3 in, 3 out]
                                n291 = invoke on="Output3-Potential Difference" class="XYGraph (strict)" method="Reinit To Default"() -> ()  [unwired: 3 in, 3 out]
                                n292 = invoke on="Output1-Time" class="XYGraph (strict)" method="Reinit To Default"() -> ()  [unwired: 3 in, 3 out]
                                n293 = invoke on="Output2-Time" class="XYGraph (strict)" method="Reinit To Default"() -> ()  [unwired: 3 in, 3 out]
                                n294 = invoke on="Output3-Time" class="XYGraph (strict)" method="Reinit To Default"() -> ()  [unwired: 3 in, 3 out]
                                n295 = invoke on="Potential Difference-Time" class="XYGraph (strict)" method="Reinit To Default"() -> ()  [unwired: 3 in, 3 out]
                              }
                              frame #1 {
                                n296 = property on="Output2-Potential Difference" class="XYGraph (strict)"("Value"=w942) -> ()  [unwired: 2 in, 2 out]
                                n297 = property on="Output1-Potential Difference" class="XYGraph (strict)"("Value"=w941) -> ()  [unwired: 2 in, 2 out]
                                n298 = property on="Output3-Potential Difference" class="XYGraph (strict)"("Value"=w943) -> ()  [unwired: 2 in, 2 out]
                                n299 = property on="Output1-Time" class="XYGraph (strict)"("Value"=w944) -> ()  [unwired: 2 in, 2 out]
                                n300 = property on="Output2-Time" class="XYGraph (strict)"("Value"=w945) -> ()  [unwired: 2 in, 2 out]
                                n301 = property on="Potential Difference-Time" class="XYGraph (strict)"("Value"=w947) -> ()  [unwired: 2 in, 2 out]
                                n302 = property on="Output3-Time" class="XYGraph (strict)"("Value"=w946) -> ()  [unwired: 2 in, 2 out]
                              }
                            }
                          }
                        }
                      }
                      frame True {
                        # "Make Aux Offset \nOpposite to Sine Out"
                        # "Sine Voltage"
                        # "Aux Voltage"
                        n303 = Divide(x=w1129, y=2) -> (x/y=w1138:dbl)
                        n304 = Divide(x=w1129, y=2) -> (x/y=w1131:dbl)
                        n305 = To Long Integer(number=w1138) -> (32bit integer=w1125:i32)
                        n306 = To Long Integer(number=w1131) -> (32bit integer=w1123:i32)
                        n307 = Subtract(x=w1136, y=w1134) -> (x-y=w1137:dbl)
                        n308 = Decrement(x=w1125) -> (x-1=w1124:i32)
                        n309 = Greater?(x=w1124, y=w1135) -> (0:w1140:bool)
                        n310 = Subtract(x=w1126, y=w1127) -> (x-y=w1130:dbl)
                        n311 = Decrement(x=w1123) -> (x-1=w1122:i32)
                        n312 = Greater?(x=w1122, y=w1128) -> (0:w1133:bool)
                        n313 = case shown="False" w1140 {
                          tunnel: [w1261 w1267] -> w1092
                          tunnel: w1124 -> [w1265 w1273]
                          tunnel: w1137 -> [w1264 w1272]
                          tunnel: w1136 -> [_ w1271]
                          tunnel: w1135 -> [w1266 w1268]
                          tunnel: w1129 -> [w1256 _]
                          tunnel: w1134 -> [w1262 _]
                          frame False {
                            n314 = Decrement(x=w1256) -> (x-1=w1257:i32)
                            n315 = Subtract(x=w1257, y=w1265) -> (x-y=w1263:i32)
                            n316 = Subtract(x=w1266, y=w1265) -> (x-y=w1259:i32)
                            n317 = Divide(x=w1264, y=w1263) -> (x/y=w1260:dbl)
                            n318 = Multiply(x=w1259, y=w1260) -> (x*y=w1258:dbl)
                            n319 = Add(x=w1258, y=w1262) -> (x+y=w1261:dbl)
                          }
                          frame True {
                            n320 = Divide(x=w1272, y=w1273) -> (x/y=w1269:dbl)
                            n321 = Multiply(x=w1268, y=w1269) -> (x*y=w1270:dbl)
                            n322 = Subtract(x=w1271, y=w1270) -> (x-y=w1267:dbl)
                          }
                        }
                        n323 = case shown="False" w1133 {
                          tunnel: [w1243 w1249] -> w1093
                          tunnel: w1122 -> [w1247 w1255]
                          tunnel: w1130 -> [w1246 w1254]
                          tunnel: w1126 -> [_ w1253]
                          tunnel: w1128 -> [w1248 w1250]
                          tunnel: w1129 -> [w1239 _]
                          tunnel: w1127 -> [w1244 _]
                          frame False {
                            n324 = Decrement(x=w1239) -> (x-1=w1238:i32)
                            n325 = Subtract(x=w1248, y=w1247) -> (x-y=w1241:i32)
                            n326 = Subtract(x=w1238, y=w1247) -> (x-y=w1245:i32)
                            n327 = Divide(x=w1246, y=w1245) -> (x/y=w1242:dbl)
                            n328 = Multiply(x=w1241, y=w1242) -> (x*y=w1240:dbl)
                            n329 = Add(x=w1240, y=w1244) -> (x+y=w1243:dbl)
                          }
                          frame True {
                            n330 = Divide(x=w1254, y=w1255) -> (x/y=w1251:dbl)
                            n331 = Multiply(x=w1250, y=w1251) -> (x*y=w1252:dbl)
                            n332 = Subtract(x=w1253, y=w1252) -> (x-y=w1249:dbl)
                          }
                        }
                        n333 = Add(x=w1102, y=w1104) -> (x+y=w1111:dbl)
                        n334 = Add(x=w1101, y=w1111) -> (x+y=w1109:dbl)
                        n335 = Negate(x=w1093) -> (-x=w1108:dbl)
                        n336 = Add(x=w1109, y=w1103) -> (x+y=w1110:dbl)
                        n337 = while {
                          tunnel: w1108 -> [w1209]
                          tunnel: w1110 -> [w1181]
                          tunnel: w1092 -> [w1208]
                          shift-right: [w1180] -> _
                          shift-left: FALSE -> [w1207]
                          tunnel: w1096 -> [w1203]
                          tunnel: w1097 -> [w1202]
                          tunnel: [w1193] -> w1094
                          tunnel: [w1192] -> w1095
                          tunnel: w1099 -> [w1199]
                          tunnel: w1100 -> [w1196]
                          tunnel: w1106 -> [w1191]
                          tunnel: w1107 -> [w1190]
                          tunnel: w1098 -> [w1189]
                          shift-right: [w1176] -> _
                          shift-left: FALSE -> [w1184]
                          shift-right: [w1177] -> _
                          shift-left: FALSE -> [w1186]
                          tunnel: w1102 -> [w1187]
                          tunnel: w1111 -> [w1183]
                          tunnel: w1109 -> [w1182]
                          shift-right: [w1172] -> w1076
                          shift-left: w1091 -> [w1169]
                          shift-right: [w1171] -> w1075
                          shift-left: w1090 -> [w1168]
                          shift-right: [w1170] -> w1074
                          shift-left: w1089 -> [w1167]
                          tunnel: w1105 -> [w1162]
                          shift-right: [w1159] -> w1077
                          shift-left: w1088 -> [w1158]
                          shift-right: [w1155] -> w1078
                          shift-left: w1087 -> [w1157]
                          tunnel: w1086 -> [w1156]
                          stop <- w1188 stop-if-true
                          # "Offset Potential\nDifference"
                          # "0V Intermission"
                          # "Bias Intermission"
                          # "0V Time"
                          # "Bias Time"
                          n338 = feedback #4() -> (w1188:bool)  [unwired: 1 in]
                          n339 = call "Elapsed Time4"("Time Target (s)"=w1183, "Reset"=w1188) -> ("Time has Elapsed"=w1206:bool)  [unwired: 10 in, 7 out]
                          n340 = call "Elapsed Time5"("Time Target (s)"=w1181, "Reset"=w1188) -> ("Time has Elapsed"=w1204:bool)  [unwired: 10 in, 7 out]
                          n341 = call "Elapsed Time16"("Time Target (s)"=w1187, "Reset"=w1188) -> ("Time has Elapsed"=w1179:bool)  [unwired: 10 in, 7 out]
                          n342 = Or(x=w1207, y=w1206) -> (x .or. y?=w1180:bool)
                          n343 = Or(x=w1186, y=w1179) -> (x .or. y?=w1177:bool)
                          n344 = case shown="False" w1180 {
                            tunnel: [w1232 0.0] -> w1174
                            tunnel: [w1234 0.0] -> w1173
                            tunnel: w1209 -> [w1234 _]
                            tunnel: [FALSE ("Time has Elapsed") w1235] -> w1205
                            tunnel: w1208 -> [w1232 _]
                            tunnel: w1204 -> [_ w1235]
                            frame False {
                            }
                            frame True {
                            }
                          }
                          n345 = call "Elapsed Time17"("Time Target (s)"=w1182, "Reset"=w1188) -> ("Time has Elapsed"=w1185:bool)  [unwired: 10 in, 7 out]
                          n346 = feedback-in #4(w1205) -> ()
                          n347 = Or(x=w1184, y=w1185) -> (x .or. y?=w1176:bool)
                          n348 = Not(x=w1180) -> (.not. x?=w1178:bool)
                          n349 = And(x=w1177, y=w1178) -> (x .and. y?=w1175:bool)
                          n350 = Or(x=w1176, y=w1175) -> (x .or. y?=w1163:bool)
                          n351 = Subtract(x=w1174, y=w1173) -> (x-y=w1164:dbl)
                          n352 = call <instrlib>:"Configure Aux Output.vi"("error in (no error)"=w1202, "Aux Output Voltage (0)"=w1173, "Aux Channel (1: Channel 1)"=w1189, "VISA resource name"=w1203) -> ("error out"=w1200:errorcluster, "VISA resource name out"=w1201:refnum<visa-resource-name>)  [unwired: 6 in]
                          n353 = call <instrlib>:"Configure Sine Out.vi"("error in (no error)"=w1200, "Sine Out DC Level to Voltage (0 V)"=w1174, "Sine Out Amplitude to Voltage (0 V)"=w1199, "VISA resource name"=w1201) -> ("error out"=w1197:errorcluster, "VISA resource name out"=w1198:refnum<visa-resource-name>)  [unwired: 6 in]
                          n354 = call <instrlib>:"Configure Reference.vi"("VISA resource name"=w1198, "Internal Reference Frequency (100000Hz)"=w1196, "error in (no error)"=w1197) -> ("VISA resource name out"=w1195:refnum<visa-resource-name>, "error out"=w1194:errorcluster)  [unwired: 11 in]
                          n355 = call <instrlib>:"Read Multiple Parameters.vi"("Single Lock-in Parameter 3 (-1: None)"=w1162, "error in (no error)"=w1194, "Single Lock-in Parameter 2 (0: X output)"=w1190, "Single Lock-in Parameter 1 (0: X output)"=w1191, "VISA resource name"=w1195) -> ("error out"=w1192:errorcluster, "Output Value(3 parameters)"=w1161:T1, "VISA resource name out"=w1193:refnum<visa-resource-name>)  [unwired: 3 in, 1 out]
                          n356 = Unbundle(w1161) -> ("Value 1"=w1166:dbl, "Value 2"=w1165:dbl, "Value 3"=w1160:dbl)
                          n357 = case shown="True" w1163 {
                            tunnel: [w1214 w1231] -> w1172
                            tunnel: [w1213 w1230] -> w1171
                            tunnel: [w1212 w1229] -> w1170
                            tunnel: w1169 -> [w1214 w1228]
                            tunnel: w1168 -> [w1213 w1227]
                            tunnel: w1167 -> [w1212 w1226]
                            tunnel: w1166 -> [_ w1219]
                            tunnel: w1165 -> [_ w1220]
                            tunnel: w1164 -> [_ w1222]
                            tunnel: w1160 -> [_ w1221]
                            tunnel: [w1211 w1225] -> w1159
                            tunnel: [w1210 w1224] -> w1155
                            tunnel: w1158 -> [w1211 w1223]
                            tunnel: w1157 -> [w1210 w1218]
                            tunnel: w1156 -> [_ w1217]
                            frame False {
                            }
                            frame True {
                              n358 = call <vilib>:"High Resolution Relative Seconds.vi"() -> ("relative seconds"=w1216:dbl)
                              n359 = Subtract(x=w1216, y=w1217) -> (x-y=w1215:dbl)
                              n360 = Build Array (concatenate)(w1228, w1219) -> (w1231:dbl[])
                              n361 = Build Array (concatenate)(w1227, w1220) -> (w1230:dbl[])
                              n362 = Build Array (concatenate)(w1226, w1221) -> (w1229:dbl[])
                              n363 = Build Array (concatenate)(w1223, w1222) -> (w1225:dbl[])
                              n364 = Build Array (concatenate)(w1218, w1215) -> (w1224:dbl[])
                            }
                          }
                        }
                        n365 = Bundle(w1077, w1075) -> (w1084:cluster{dbl[], dbl[]})  [unwired: 1 in]
                        n366 = Bundle(w1077, w1074) -> (w1085:cluster{dbl[], dbl[]})  [unwired: 1 in]
                        n367 = Bundle(w1078, w1076) -> (w1082:cluster{dbl[], dbl[]})  [unwired: 1 in]
                        n368 = Bundle(w1077, w1076) -> (w1083:cluster{dbl[], dbl[]})  [unwired: 1 in]
                        n369 = Bundle(w1078, w1074) -> (w1080:cluster{dbl[], dbl[]})  [unwired: 1 in]
                        n370 = Bundle(w1078, w1075) -> (w1081:cluster{dbl[], dbl[]})  [unwired: 1 in]
                        n371 = Bundle(w1078, w1077) -> (w1079:cluster{dbl[], dbl[]})  [unwired: 1 in]
                        n372 = flat-sequence {
                          tunnel: [w1147] -> w1121
                          tunnel: w1083 -> [w1147]
                          tunnel: [w1146] -> w1120
                          tunnel: w1084 -> [w1146]
                          tunnel: w1079 -> [w1145]
                          tunnel: [w1145] -> w1119
                          tunnel: w1080 -> [w1144]
                          tunnel: [w1144] -> w1118
                          tunnel: w1081 -> [w1143]
                          tunnel: [w1143] -> w1117
                          tunnel: w1085 -> [w1142]
                          tunnel: [w1142] -> w1116
                          tunnel: w1082 -> [w1141]
                          tunnel: [w1141] -> w1115
                          tunnel: w1121 -> [w1148]
                          tunnel: w1120 -> [w1149]
                          tunnel: w1119 -> [w1154]
                          tunnel: w1118 -> [w1153]
                          tunnel: w1117 -> [w1152]
                          tunnel: w1116 -> [w1150]
                          tunnel: w1115 -> [w1151]
                          tunnel: [w1154] -> w1073
                          tunnel: [w1153] -> w1072
                          tunnel: [w1152] -> w1071
                          tunnel: [w1151] -> w1070
                          tunnel: [w1150] -> w1069
                          tunnel: [w1149] -> w1068
                          tunnel: [w1148] -> w1067
                          frame #0 {
                            n373 = invoke on="Output3-Potential Difference" class="XYGraph (strict)" method="Reinit To Default"() -> ()  [unwired: 3 in, 3 out]
                            n374 = invoke on="Output1-Time" class="XYGraph (strict)" method="Reinit To Default"() -> ()  [unwired: 3 in, 3 out]
                            n375 = invoke on="Potential Difference-Time" class="XYGraph (strict)" method="Reinit To Default"() -> ()  [unwired: 3 in, 3 out]
                            n376 = invoke on="Output2-Potential Difference" class="XYGraph (strict)" method="Reinit To Default"() -> ()  [unwired: 3 in, 3 out]
                            n377 = invoke on="Output1-Potential Difference" class="XYGraph (strict)" method="Reinit To Default"() -> ()  [unwired: 3 in, 3 out]
                            n378 = invoke on="Output3-Time" class="XYGraph (strict)" method="Reinit To Default"() -> ()  [unwired: 3 in, 3 out]
                            n379 = invoke on="Output2-Time" class="XYGraph (strict)" method="Reinit To Default"() -> ()  [unwired: 3 in, 3 out]
                          }
                          frame #1 {
                            n380 = property on="Output1-Time" class="XYGraph (strict)"("Value"=w1151) -> ()  [unwired: 2 in, 2 out]
                            n381 = property on="Potential Difference-Time" class="XYGraph (strict)"("Value"=w1154) -> ()  [unwired: 2 in, 2 out]
                            n382 = property on="Output2-Potential Difference" class="XYGraph (strict)"("Value"=w1149) -> ()  [unwired: 2 in, 2 out]
                            n383 = property on="Output3-Potential Difference" class="XYGraph (strict)"("Value"=w1150) -> ()  [unwired: 2 in, 2 out]
                            n384 = property on="Output2-Time" class="XYGraph (strict)"("Value"=w1152) -> ()  [unwired: 2 in, 2 out]
                            n385 = property on="Output3-Time" class="XYGraph (strict)"("Value"=w1153) -> ()  [unwired: 2 in, 2 out]
                            n386 = property on="Output1-Potential Difference" class="XYGraph (strict)"("Value"=w1148) -> ()  [unwired: 2 in, 2 out]
                          }
                        }
                      }
                    }
                  }
                  frame True {
                    # "Make Aux Offset \nOpposite to Sine Out"
                    # "Sine\nVoltage"
                    # "Aux\nVoltage"
                    n387 = Multiply(x=w1335, y=w1336) -> (x*y=w1334:dbl)
                    n388 = Multiply(x=w1331, y=w1330) -> (x*y=w1332:dbl)
                    n389 = Subtract(x=w1333, y=w1334) -> (x-y=w1299:dbl)
                    n390 = Subtract(x=w1329, y=w1332) -> (x-y=w1302:dbl)
                    n391 = Add(x=w1303, y=w1301) -> (x+y=w1318:dbl)
                    n392 = Add(x=w1304, y=w1318) -> (x+y=w1316:dbl)
                    n393 = Negate(x=w1299) -> (-x=w1315:dbl)
                    n394 = Add(x=w1316, y=w1300) -> (x+y=w1317:dbl)
                    n395 = while {
                      tunnel: w1315 -> [w1405]
                      tunnel: w1317 -> [w1377]
                      tunnel: w1302 -> [w1404]
                      shift-right: [w1376] -> _
                      shift-left: FALSE -> [w1403]
                      tunnel: w1313 -> [w1399]
                      tunnel: w1314 -> [w1398]
                      tunnel: [w1389] -> w1306
                      tunnel: [w1388] -> w1307
                      tunnel: w1312 -> [w1395]
                      tunnel: w1311 -> [w1392]
                      tunnel: w1309 -> [w1387]
                      tunnel: w1308 -> [w1386]
                      tunnel: w1305 -> [w1385]
                      shift-right: [w1372] -> _
                      shift-left: FALSE -> [w1380]
                      shift-right: [w1373] -> _
                      shift-left: FALSE -> [w1382]
                      tunnel: w1303 -> [w1383]
                      tunnel: w1318 -> [w1379]
                      tunnel: w1316 -> [w1378]
                      shift-right: [w1368] -> w1284
                      shift-left: w1294 -> [w1365]
                      shift-right: [w1367] -> w1283
                      shift-left: w1295 -> [w1364]
                      shift-right: [w1366] -> w1282
                      shift-left: w1296 -> [w1363]
                      tunnel: w1310 -> [w1358]
                      shift-right: [w1355] -> w1286
                      shift-left: w1297 -> [w1354]
                      shift-right: [w1352] -> w1285
                      shift-left: w1298 -> [w1353]
                      tunnel: w1281 -> [w1351]
                      stop <- w1384 stop-if-true
                      # "Offset Potential\nDifference"
                      # "0V Intermission"
                      # "Bias Intermission"
                      # "0V Time"
                      # "Bias Time"
                      n396 = feedback #5() -> (w1384:bool)  [unwired: 1 in]
                      n397 = call "Elapsed Time2"("Time Target (s)"=w1379, "Reset"=w1384) -> ("Time has Elapsed"=w1402:bool)  [unwired: 10 in, 7 out]
                      n398 = call "Elapsed Time3"("Time Target (s)"=w1377, "Reset"=w1384) -> ("Time has Elapsed"=w1400:bool)  [unwired: 10 in, 7 out]
                      n399 = call "Elapsed Time14"("Time Target (s)"=w1383, "Reset"=w1384) -> ("Time has Elapsed"=w1375:bool)  [unwired: 10 in, 7 out]
                      n400 = Or(x=w1403, y=w1402) -> (x .or. y?=w1376:bool)
                      n401 = Or(x=w1382, y=w1375) -> (x .or. y?=w1373:bool)
                      n402 = case shown="False" w1376 {
                        tunnel: [w1428 0.0] -> w1370
                        tunnel: [w1430 0.0] -> w1369
                        tunnel: w1405 -> [w1430 _]
                        tunnel: [FALSE ("Time has Elapsed") w1431] -> w1401
                        tunnel: w1404 -> [w1428 _]
                        tunnel: w1400 -> [_ w1431]
                        frame False {
                        }
                        frame True {
                        }
                      }
                      n403 = call "Elapsed Time15"("Time Target (s)"=w1378, "Reset"=w1384) -> ("Time has Elapsed"=w1381:bool)  [unwired: 10 in, 7 out]
                      n404 = feedback-in #5(w1401) -> ()
                      n405 = Or(x=w1380, y=w1381) -> (x .or. y?=w1372:bool)
                      n406 = Not(x=w1376) -> (.not. x?=w1374:bool)
                      n407 = And(x=w1373, y=w1374) -> (x .and. y?=w1371:bool)
                      n408 = Or(x=w1372, y=w1371) -> (x .or. y?=w1359:bool)
                      n409 = Subtract(x=w1370, y=w1369) -> (x-y=w1360:dbl)
                      n410 = call <instrlib>:"Configure Aux Output.vi"("error in (no error)"=w1398, "Aux Output Voltage (0)"=w1369, "Aux Channel (1: Channel 1)"=w1385, "VISA resource name"=w1399) -> ("error out"=w1396:errorcluster, "VISA resource name out"=w1397:refnum<visa-resource-name>)  [unwired: 6 in]
                      n411 = call <instrlib>:"Configure Sine Out.vi"("error in (no error)"=w1396, "Sine Out DC Level to Voltage (0 V)"=w1370, "Sine Out Amplitude to Voltage (0 V)"=w1395, "VISA resource name"=w1397) -> ("error out"=w1393:errorcluster, "VISA resource name out"=w1394:refnum<visa-resource-name>)  [unwired: 6 in]
                      n412 = call <instrlib>:"Configure Reference.vi"("VISA resource name"=w1394, "Internal Reference Frequency (100000Hz)"=w1392, "error in (no error)"=w1393) -> ("VISA resource name out"=w1391:refnum<visa-resource-name>, "error out"=w1390:errorcluster)  [unwired: 11 in]
                      n413 = call <instrlib>:"Read Multiple Parameters.vi"("Single Lock-in Parameter 3 (-1: None)"=w1358, "error in (no error)"=w1390, "Single Lock-in Parameter 2 (0: X output)"=w1386, "Single Lock-in Parameter 1 (0: X output)"=w1387, "VISA resource name"=w1391) -> ("error out"=w1388:errorcluster, "Output Value(3 parameters)"=w1357:T1, "VISA resource name out"=w1389:refnum<visa-resource-name>)  [unwired: 3 in, 1 out]
                      n414 = Unbundle(w1357) -> ("Value 1"=w1362:dbl, "Value 2"=w1361:dbl, "Value 3"=w1356:dbl)
                      n415 = case shown="True" w1359 {
                        tunnel: [w1410 w1427] -> w1368
                        tunnel: [w1409 w1426] -> w1367
                        tunnel: [w1408 w1425] -> w1366
                        tunnel: w1365 -> [w1410 w1424]
                        tunnel: w1364 -> [w1409 w1423]
                        tunnel: w1363 -> [w1408 w1422]
                        tunnel: w1362 -> [_ w1415]
                        tunnel: w1361 -> [_ w1416]
                        tunnel: w1360 -> [_ w1418]
                        tunnel: w1356 -> [_ w1417]
                        tunnel: [w1407 w1421] -> w1355
                        tunnel: [w1406 w1420] -> w1352
                        tunnel: w1354 -> [w1407 w1419]
                        tunnel: w1353 -> [w1406 w1414]
                        tunnel: w1351 -> [_ w1413]
                        frame False {
                        }
                        frame True {
                          n416 = call <vilib>:"High Resolution Relative Seconds.vi"() -> ("relative seconds"=w1412:dbl)
                          n417 = Subtract(x=w1412, y=w1413) -> (x-y=w1411:dbl)
                          n418 = Build Array (concatenate)(w1424, w1415) -> (w1427:dbl[])
                          n419 = Build Array (concatenate)(w1423, w1416) -> (w1426:dbl[])
                          n420 = Build Array (concatenate)(w1422, w1417) -> (w1425:dbl[])
                          n421 = Build Array (concatenate)(w1419, w1418) -> (w1421:dbl[])
                          n422 = Build Array (concatenate)(w1414, w1411) -> (w1420:dbl[])
                        }
                      }
                    }
                    n423 = Bundle(w1286, w1283) -> (w1292:cluster{dbl[], dbl[]})  [unwired: 1 in]
                    n424 = Bundle(w1286, w1282) -> (w1291:cluster{dbl[], dbl[]})  [unwired: 1 in]
                    n425 = Bundle(w1285, w1286) -> (w1287:cluster{dbl[], dbl[]})  [unwired: 1 in]
                    n426 = Bundle(w1286, w1284) -> (w1293:cluster{dbl[], dbl[]})  [unwired: 1 in]
                    n427 = Bundle(w1285, w1284) -> (w1290:cluster{dbl[], dbl[]})  [unwired: 1 in]
                    n428 = Bundle(w1285, w1282) -> (w1288:cluster{dbl[], dbl[]})  [unwired: 1 in]
                    n429 = Bundle(w1285, w1283) -> (w1289:cluster{dbl[], dbl[]})  [unwired: 1 in]
                    n430 = flat-sequence {
                      tunnel: [w1343] -> w1328
                      tunnel: w1293 -> [w1343]
                      tunnel: [w1342] -> w1327
                      tunnel: w1292 -> [w1342]
                      tunnel: w1287 -> [w1341]
                      tunnel: [w1341] -> w1326
                      tunnel: w1288 -> [w1340]
                      tunnel: [w1340] -> w1325
                      tunnel: w1289 -> [w1339]
                      tunnel: [w1339] -> w1324
                      tunnel: w1291 -> [w1338]
                      tunnel: [w1338] -> w1323
                      tunnel: w1290 -> [w1337]
                      tunnel: [w1337] -> w1322
                      tunnel: w1328 -> [w1344]
                      tunnel: w1327 -> [w1345]
                      tunnel: w1326 -> [w1350]
                      tunnel: w1325 -> [w1349]
                      tunnel: w1324 -> [w1348]
                      tunnel: w1323 -> [w1346]
                      tunnel: w1322 -> [w1347]
                      tunnel: [w1350] -> w1280
                      tunnel: [w1349] -> w1279
                      tunnel: [w1348] -> w1278
                      tunnel: [w1347] -> w1277
                      tunnel: [w1346] -> w1276
                      tunnel: [w1345] -> w1275
                      tunnel: [w1344] -> w1274
                      frame #0 {
                        n431 = invoke on="Output2-Potential Difference" class="XYGraph (strict)" method="Reinit To Default"() -> ()  [unwired: 3 in, 3 out]
                        n432 = invoke on="Output1-Potential Difference" class="XYGraph (strict)" method="Reinit To Default"() -> ()  [unwired: 3 in, 3 out]
                        n433 = invoke on="Output1-Time" class="XYGraph (strict)" method="Reinit To Default"() -> ()  [unwired: 3 in, 3 out]
                        n434 = invoke on="Output3-Potential Difference" class="XYGraph (strict)" method="Reinit To Default"() -> ()  [unwired: 3 in, 3 out]
                        n435 = invoke on="Potential Difference-Time" class="XYGraph (strict)" method="Reinit To Default"() -> ()  [unwired: 3 in, 3 out]
                        n436 = invoke on="Output2-Time" class="XYGraph (strict)" method="Reinit To Default"() -> ()  [unwired: 3 in, 3 out]
                        n437 = invoke on="Output3-Time" class="XYGraph (strict)" method="Reinit To Default"() -> ()  [unwired: 3 in, 3 out]
                      }
                      frame #1 {
                        n438 = property on="Output3-Potential Difference" class="XYGraph (strict)"("Value"=w1346) -> ()  [unwired: 2 in, 2 out]
                        n439 = property on="Potential Difference-Time" class="XYGraph (strict)"("Value"=w1350) -> ()  [unwired: 2 in, 2 out]
                        n440 = property on="Output2-Time" class="XYGraph (strict)"("Value"=w1348) -> ()  [unwired: 2 in, 2 out]
                        n441 = property on="Output3-Time" class="XYGraph (strict)"("Value"=w1349) -> ()  [unwired: 2 in, 2 out]
                        n442 = property on="Output1-Potential Difference" class="XYGraph (strict)"("Value"=w1344) -> ()  [unwired: 2 in, 2 out]
                        n443 = property on="Output2-Potential Difference" class="XYGraph (strict)"("Value"=w1345) -> ()  [unwired: 2 in, 2 out]
                        n444 = property on="Output1-Time" class="XYGraph (strict)"("Value"=w1347) -> ()  [unwired: 2 in, 2 out]
                      }
                    }
                  }
                }
              }
              frame True {
                # "Make Aux Offset \nOpposite to Sine Out"
                # "Sine\nVoltage"
                # "Aux\nVoltage"
                n445 = Multiply(x=w1493, y=w1496) -> (x*y=w1495:dbl)
                n446 = Multiply(x=w1491, y=w1490) -> (x*y=w1492:dbl)
                n447 = Add(x=w1495, y=w1494) -> (x+y=w1447:dbl)
                n448 = Add(x=w1492, y=w1489) -> (x+y=w1455:dbl)
                n449 = Add(x=w1456, y=w1453) -> (x+y=w1478:dbl)
                n450 = Add(x=w1457, y=w1478) -> (x+y=w1476:dbl)
                n451 = Negate(x=w1447) -> (-x=w1475:dbl)
                n452 = Add(x=w1476, y=w1454) -> (x+y=w1477:dbl)
                n453 = while {
                  tunnel: w1475 -> [w1565]
                  tunnel: w1477 -> [w1537]
                  tunnel: w1455 -> [w1564]
                  shift-right: [w1536] -> _
                  shift-left: FALSE -> [w1563]
                  tunnel: w1461 -> [w1559]
                  tunnel: w1462 -> [w1558]
                  tunnel: [w1549] -> w1467
                  tunnel: [w1548] -> w1466
                  tunnel: w1464 -> [w1555]
                  tunnel: w1465 -> [w1552]
                  tunnel: w1459 -> [w1547]
                  tunnel: w1458 -> [w1546]
                  tunnel: w1463 -> [w1545]
                  shift-right: [w1532] -> _
                  shift-left: FALSE -> [w1540]
                  shift-right: [w1533] -> _
                  shift-left: FALSE -> [w1542]
                  tunnel: w1456 -> [w1543]
                  tunnel: w1478 -> [w1539]
                  tunnel: w1476 -> [w1538]
                  shift-right: [w1528] -> w1442
                  shift-left: w1448 -> [w1525]
                  shift-right: [w1527] -> w1441
                  shift-left: w1449 -> [w1524]
                  shift-right: [w1526] -> w1443
                  shift-left: w1450 -> [w1523]
                  tunnel: w1460 -> [w1518]
                  shift-right: [w1515] -> w1444
                  shift-left: w1451 -> [w1513]
                  shift-right: [w1514] -> w1445
                  shift-left: w1452 -> [w1512]
                  tunnel: w1446 -> [w1511]
                  stop <- w1544 stop-if-true
                  # "Offset Potential\nDifference"
                  # "0V Intermission"
                  # "Bias Intermission"
                  # "0V Time"
                  # "Bias Time"
                  n454 = feedback #6() -> (w1544:bool)  [unwired: 1 in]
                  n455 = call "Elapsed Time"("Time Target (s)"=w1539, "Reset"=w1544) -> ("Time has Elapsed"=w1562:bool)  [unwired: 10 in, 7 out]
                  n456 = call "Elapsed Time12"("Time Target (s)"=w1537, "Reset"=w1544) -> ("Time has Elapsed"=w1560:bool)  [unwired: 10 in, 7 out]
                  n457 = call "Elapsed Time13"("Time Target (s)"=w1543, "Reset"=w1544) -> ("Time has Elapsed"=w1535:bool)  [unwired: 10 in, 7 out]
                  n458 = Or(x=w1563, y=w1562) -> (x .or. y?=w1536:bool)
                  n459 = Or(x=w1542, y=w1535) -> (x .or. y?=w1533:bool)
                  n460 = case shown="False" w1536 {
                    tunnel: [w1588 0.0] -> w1530
                    tunnel: [w1590 0.0] -> w1529
                    tunnel: w1565 -> [w1590 _]
                    tunnel: [FALSE ("Time has Elapsed") w1591] -> w1561
                    tunnel: w1564 -> [w1588 _]
                    tunnel: w1560 -> [_ w1591]
                    frame False {
                    }
                    frame True {
                    }
                  }
                  n461 = call "Elapsed Time24"("Time Target (s)"=w1538, "Reset"=w1544) -> ("Time has Elapsed"=w1541:bool)  [unwired: 10 in, 7 out]
                  n462 = feedback-in #6(w1561) -> ()
                  n463 = Or(x=w1540, y=w1541) -> (x .or. y?=w1532:bool)
                  n464 = Not(x=w1536) -> (.not. x?=w1534:bool)
                  n465 = And(x=w1533, y=w1534) -> (x .and. y?=w1531:bool)
                  n466 = Or(x=w1532, y=w1531) -> (x .or. y?=w1519:bool)
                  n467 = Subtract(x=w1530, y=w1529) -> (x-y=w1520:dbl)
                  n468 = call <instrlib>:"Configure Aux Output.vi"("error in (no error)"=w1558, "Aux Output Voltage (0)"=w1529, "Aux Channel (1: Channel 1)"=w1545, "VISA resource name"=w1559) -> ("error out"=w1556:errorcluster, "VISA resource name out"=w1557:refnum<visa-resource-name>)  [unwired: 6 in]
                  n469 = call <instrlib>:"Configure Sine Out.vi"("error in (no error)"=w1556, "Sine Out DC Level to Voltage (0 V)"=w1530, "Sine Out Amplitude to Voltage (0 V)"=w1555, "VISA resource name"=w1557) -> ("error out"=w1553:errorcluster, "VISA resource name out"=w1554:refnum<visa-resource-name>)  [unwired: 6 in]
                  n470 = call <instrlib>:"Configure Reference.vi"("VISA resource name"=w1554, "Internal Reference Frequency (100000Hz)"=w1552, "error in (no error)"=w1553) -> ("VISA resource name out"=w1551:refnum<visa-resource-name>, "error out"=w1550:errorcluster)  [unwired: 11 in]
                  n471 = call <instrlib>:"Read Multiple Parameters.vi"("Single Lock-in Parameter 3 (-1: None)"=w1518, "error in (no error)"=w1550, "Single Lock-in Parameter 2 (0: X output)"=w1546, "Single Lock-in Parameter 1 (0: X output)"=w1547, "VISA resource name"=w1551) -> ("error out"=w1548:errorcluster, "Output Value(3 parameters)"=w1517:T1, "VISA resource name out"=w1549:refnum<visa-resource-name>)  [unwired: 3 in, 1 out]
                  n472 = Unbundle(w1517) -> ("Value 1"=w1522:dbl, "Value 2"=w1521:dbl, "Value 3"=w1516:dbl)
                  n473 = case shown="True" w1519 {
                    tunnel: [w1570 w1587] -> w1528
                    tunnel: [w1569 w1586] -> w1527
                    tunnel: [w1568 w1585] -> w1526
                    tunnel: w1525 -> [w1570 w1584]
                    tunnel: w1524 -> [w1569 w1583]
                    tunnel: w1523 -> [w1568 w1582]
                    tunnel: w1522 -> [_ w1575]
                    tunnel: w1521 -> [_ w1576]
                    tunnel: w1520 -> [_ w1578]
                    tunnel: w1516 -> [_ w1577]
                    tunnel: [w1567 w1581] -> w1515
                    tunnel: [w1566 w1580] -> w1514
                    tunnel: w1513 -> [w1567 w1579]
                    tunnel: w1512 -> [w1566 w1574]
                    tunnel: w1511 -> [_ w1572]
                    frame False {
                    }
                    frame True {
                      n474 = call <vilib>:"High Resolution Relative Seconds.vi"() -> ("relative seconds"=w1573:dbl)
                      n475 = Subtract(x=w1573, y=w1572) -> (x-y=w1571:dbl)
                      n476 = Build Array (concatenate)(w1584, w1575) -> (w1587:dbl[])
                      n477 = Build Array (concatenate)(w1583, w1576) -> (w1586:dbl[])
                      n478 = Build Array (concatenate)(w1582, w1577) -> (w1585:dbl[])
                      n479 = Build Array (concatenate)(w1579, w1578) -> (w1581:dbl[])
                      n480 = Build Array (concatenate)(w1574, w1571) -> (w1580:dbl[])
                    }
                  }
                }
                n481 = Bundle(w1444, w1441) -> (w1470:cluster{dbl[], dbl[]})  [unwired: 1 in]
                n482 = Bundle(w1444, w1443) -> (w1471:cluster{dbl[], dbl[]})  [unwired: 1 in]
                n483 = Bundle(w1445, w1442) -> (w1472:cluster{dbl[], dbl[]})  [unwired: 1 in]
                n484 = Bundle(w1444, w1442) -> (w1469:cluster{dbl[], dbl[]})  [unwired: 1 in]
                n485 = Bundle(w1445, w1443) -> (w1468:cluster{dbl[], dbl[]})  [unwired: 1 in]
                n486 = Bundle(w1445, w1441) -> (w1473:cluster{dbl[], dbl[]})  [unwired: 1 in]
                n487 = Bundle(w1445, w1444) -> (w1474:cluster{dbl[], dbl[]})  [unwired: 1 in]
                n488 = flat-sequence {
                  tunnel: [w1503] -> w1488
                  tunnel: w1469 -> [w1503]
                  tunnel: [w1502] -> w1487
                  tunnel: w1470 -> [w1502]
                  tunnel: w1474 -> [w1501]
                  tunnel: [w1501] -> w1486
                  tunnel: w1468 -> [w1500]
                  tunnel: [w1500] -> w1485
                  tunnel: w1473 -> [w1499]
                  tunnel: [w1499] -> w1484
                  tunnel: w1471 -> [w1498]
                  tunnel: [w1498] -> w1483
                  tunnel: w1472 -> [w1497]
                  tunnel: [w1497] -> w1482
                  tunnel: w1488 -> [w1504]
                  tunnel: w1487 -> [w1505]
                  tunnel: w1486 -> [w1510]
                  tunnel: w1485 -> [w1509]
                  tunnel: w1484 -> [w1508]
                  tunnel: w1483 -> [w1506]
                  tunnel: w1482 -> [w1507]
                  tunnel: [w1510] -> w1440
                  tunnel: [w1509] -> w1439
                  tunnel: [w1508] -> w1438
                  tunnel: [w1507] -> w1437
                  tunnel: [w1506] -> w1436
                  tunnel: [w1505] -> w1435
                  tunnel: [w1504] -> w1434
                  frame #0 {
                    n489 = invoke on="Output1-Potential Difference" class="XYGraph (strict)" method="Reinit To Default"() -> ()  [unwired: 3 in, 3 out]
                    n490 = invoke on="Output3-Potential Difference" class="XYGraph (strict)" method="Reinit To Default"() -> ()  [unwired: 3 in, 3 out]
                    n491 = invoke on="Output2-Potential Difference" class="XYGraph (strict)" method="Reinit To Default"() -> ()  [unwired: 3 in, 3 out]
                    n492 = invoke on="Output1-Time" class="XYGraph (strict)" method="Reinit To Default"() -> ()  [unwired: 3 in, 3 out]
                    n493 = invoke on="Output2-Time" class="XYGraph (strict)" method="Reinit To Default"() -> ()  [unwired: 3 in, 3 out]
                    n494 = invoke on="Output3-Time" class="XYGraph (strict)" method="Reinit To Default"() -> ()  [unwired: 3 in, 3 out]
                    n495 = invoke on="Potential Difference-Time" class="XYGraph (strict)" method="Reinit To Default"() -> ()  [unwired: 3 in, 3 out]
                  }
                  frame #1 {
                    n496 = property on="Output2-Time" class="XYGraph (strict)"("Value"=w1508) -> ()  [unwired: 2 in, 2 out]
                    n497 = property on="Output1-Potential Difference" class="XYGraph (strict)"("Value"=w1504) -> ()  [unwired: 2 in, 2 out]
                    n498 = property on="Output2-Potential Difference" class="XYGraph (strict)"("Value"=w1505) -> ()  [unwired: 2 in, 2 out]
                    n499 = property on="Output1-Time" class="XYGraph (strict)"("Value"=w1507) -> ()  [unwired: 2 in, 2 out]
                    n500 = property on="Potential Difference-Time" class="XYGraph (strict)"("Value"=w1510) -> ()  [unwired: 2 in, 2 out]
                    n501 = property on="Output3-Potential Difference" class="XYGraph (strict)"("Value"=w1506) -> ()  [unwired: 2 in, 2 out]
                    n502 = property on="Output3-Time" class="XYGraph (strict)"("Value"=w1509) -> ()  [unwired: 2 in, 2 out]
                  }
                }
              }
            }
          }
        }
        n503 = Unbundle(w73) -> (w76:dbl[], w75:dbl[])
        n504 = Unbundle(w83) -> (w86:dbl[], w85:dbl[])
        n505 = Unbundle(w78) -> (w81:dbl[], w80:dbl[])
        n506 = Unbundle(w68) -> (w71:dbl[], w70:dbl[])
        n507 = Unbundle(w63) -> (w66:dbl[], w65:dbl[])
        n508 = Unbundle(w58) -> (w62:dbl[], w61:dbl[])
        n509 = Unbundle(w88) -> (w91:dbl[], w90:dbl[])
        n510 = Build Array(w76, w75) -> (w74:dbl[][])
        n511 = Build Array(w86, w85) -> (w84:dbl[][])
        n512 = Build Array(w81, w80) -> (w79:dbl[][])
        n513 = Build Array(w71, w70) -> (w69:dbl[][])
        n514 = Build Array(w66, w65) -> (w64:dbl[][])
        n515 = Build Array(w62, w61) -> (w60:dbl[][])
        n516 = Build Array(w91, w90) -> (w89:dbl[][])
        n517 = call-poly <vilib>:"Write Delimited Spreadsheet.vi"("file path (dialog if empty)"="Save As Path", "2D data"=w84, "transpose? (no:F)"=TRUE) -> ()  [unwired: 11 in, 2 out]
        n518 = call-poly <vilib>:"Write Delimited Spreadsheet.vi"("file path (dialog if empty)"="Save As Path", "2D data"=w79, "transpose? (no:F)"=TRUE) -> ()  [unwired: 11 in, 2 out]
        n519 = call-poly <vilib>:"Write Delimited Spreadsheet.vi"("file path (dialog if empty)"="Save As Path", "2D data"=w69, "transpose? (no:F)"=TRUE) -> ()  [unwired: 11 in, 2 out]
        n520 = call-poly <vilib>:"Write Delimited Spreadsheet.vi"("file path (dialog if empty)"="Save As Path", "2D data"=w64, "transpose? (no:F)"=TRUE) -> ()  [unwired: 11 in, 2 out]
        n521 = call-poly <vilib>:"Write Delimited Spreadsheet.vi"("file path (dialog if empty)"="Save As Path", "2D data"=w60, "transpose? (no:F)"=TRUE) -> ()  [unwired: 11 in, 2 out]
        n522 = call-poly <vilib>:"Write Delimited Spreadsheet.vi"("file path (dialog if empty)"="Save As Path", "2D data"=w89, "transpose? (no:F)"=TRUE) -> ()  [unwired: 11 in, 2 out]
        n523 = call-poly <vilib>:"Write Delimited Spreadsheet.vi"("file path (dialog if empty)"="Save As Path", "2D data"=w74, "transpose? (no:F)"=TRUE) -> ()  [unwired: 11 in, 2 out]
      }
    }
  }
  n524 = case shown="False" w2 {
    tunnel: w3 -> [w1598 w1601]
    tunnel: w4 -> [w1599 w1602]
    frame False {
      n525 = call <instrlib>:"Close.vi"("error in (no error)"=w1598, "VISA resource name"=w1599) -> ("error out"=w1600:errorcluster)  [unwired: 9 in]
      n526 = call <vilib>:"General Error Handler.vi"("error in (no error)"=w1600) -> ()  [unwired: 10 in, 5 out]
    }
    frame True {
      "VISA resource name out" <- w1602
      "error out" <- w1601
    }
  }
